vi "CPCI_fifo.vi"(10 "传递队列":refnum<queue>, 11 "notifier":refnum<notifier>) -> ()   [LabVIEW 2012]
uses:
  <vilib>/GPower/VIRegister/Library/Convert/ToBool.vi
  <vilib>/GPower/VIRegister/Library/SubVIs/FindRegisterData.vi
  <vilib>/GPower/VIRegister/Library/SubVIs/ReadSub.vi
  <vilib>/GPower/VIRegister/Library/SubVIs/WriteSub.vi
  <vilib>/GPower/VIRegister/Library/QManager/GetRegisterData.vi
  <vilib>/GPower/Error/Library/SetError.vi
  <vilib>/GPower/Error/Library/FilterCodes.vi
  <vilib>/GPower/Error/Library/Filter/FilterMulti.vi
  <vilib>/GPower/VIRegister/Library/QManager/QManagerAction.vi
  <vilib>/GPower/Error/Library/ErrorType.vi
  <vilib>/GPower/Error/Library/SplitAppended.vi
  <vilib>/GPower/Error/Library/SubVIs/ExplanationToError.vi
  <vilib>/GPower/VIRegister/Library/QManager/GetQName.vi
  <vilib>/GPower/VIRegister/Library/QManager/StartQManager.vi
  <vilib>/Utility/error.llb/Trim Whitespace.vi
  <vilib>/dlg_ctls.llb/Space Constant.vi
  <vilib>/Utility/error.llb/Error Code Database.vi
  <vilib>/GPower/Error/Library/SubVIs/SetStatus.vi
  <vilib>/GPower/Error/Library/AppendErrors.vi
  <vilib>/GPower/Error/Library/Append/AppendSingle.vi
  write32.vi
  write8.vi
  Based_on/BSCT Automation123/BSCT_BasicFunctions/BSCT_BasicFunctions.lvlib
  <vilib>/GPower/VIRegister/VIRegister.lvlib
panel:
  out "x+y 2":u32 format="%.0x"
  out "x+y":u32 format="%.0x"
  in  "8路定时配置 2":T1(array[cluster])=[[{"mode2_set"={"mode2_set01"=0, "mode2_set02"=0, "mode2_set03"=0, "mode2_set04"=0, "mode2_set05"=0, "mode2_set06"=0, "mode2_set07"=0, "mode2_set08"=0, "mode2_set09"=0, "mode2_set10"=0, "mode2_set11"=0, "mode2_set12"=0}, "mode2_t"={"mode2_t01"=0, "mode2_t02"=20, "mode2_t03"=30, "mode2_t04"=0, "mode2_t05"=0, "mode2_t06"=0, "mode2_t07"=0, "mode2_t08"=0, "mode2_t09"=0, "mode2_t10"=0, "mode2_t11"=0, "mode2_t12"=0}, "mode2_cmd_addr"={"mode2_cmd_addr01"=0, "mode2_cmd_addr02"=128, "mode2_cmd_addr03"=256, "mode2_cmd_addr04"=0, "mode2_cmd_addr05"=0, "mode2_cmd_addr06"=0, "mode2_cmd_addr07"=0, "mode2_cmd_addr08"=0, "mode2_cmd_addr09"=0, "mode2_cmd_addr10"=0, "mode2_cmd_addr11"=0, "mode2_cmd_addr12"=0}, "mode2_ cmd_len"={"mode2_ cmd_len01"=20, "mode2_ cmd_len02"=0, "mode2_ cmd_len03"=0, "mode2_ cmd_len04"=0, "mode2_ cmd_len05"=0, "mode2_ cmd_len06"=0, "mode2_ cmd_len07"=0, "mode2_ cmd_len08"=0, "mode2_ cmd_len09"=0, "mode2_ cmd_len10"=0, "mode2_ cmd_len11"=0, "mode2_ cmd_len12"=0}, "mode2_ack_addr"={"mode2_ack_addr01"=0, "mode2_ack_addr02"=128, "mode2_ack_addr03"=256, "mode2_ack_addr04"=0, "mode2_ack_addr05"=0, "mode2_ack_addr06"=0, "mode2_ack_addr07"=0, "mode2_ack_addr08"=0, "mode2_ack_addr09"=0, "mode2_ack_addr10"=0, "mode2_ack_addr11"=0, "mode2_ack_addr12"=0}, "mode2_ack_len"={"mode2_ack_len01"=0, "mode2_ack_len02"=0, "mode2_ack_len03"=0, "mode2_ack_len04"=0, "mode2_ack_len05"=0, "mode2_ack_len06"=0, "mode2_ack_len07"=0, "mode2_ack_len08"=0, "mode2_ack_len09"=0, "mode2_ack_len10"=0, "mode2_ack_len11"=0, "mode2_ack_len12"=0}, "mode2_period"={"mode2_period"=9}}, {"mode2_set"={"mode2_set01"=0, "mode2_set02"=0, "mode2_set03"=0, "mode2_set04"=0, "mode2_set05"=0, "mode2_set06"=0, "mode2_set07"=0, "mode2_set08"=0, "mode2_set09"=0, "mode2_set10"=0, "mode2_set11"=0, "mode2_set12"=0}, "mode2_t"={"mode2_t01"=0, "mode2_t02"=20, "mode2_t03"=30, "mode2_t04"=0, "mode2_t05"=0, "mode2_t06"=0, "mode2_t07"=0, "mode2_t08"=0, "mode2_t09"=0, "mode2_t10"=0, "mode2_t11"=0, "mode2_t12"=0}, "mode2_cmd_addr"={"mode2_cmd_addr01"=0, "mode2_cmd_addr02"=128, "mode2_cmd_addr03"=256, "mode2_cmd_addr04"=0, "mode2_cmd_addr05"=0, "mode2_cmd_addr06"=0, "mode2_cmd_addr07"=0, "mode2_cmd_addr08"=0, "mode2_cmd_addr09"=0, "mode2_cmd_addr10"=0, "mode2_cmd_addr11"=0, "mode2_cmd_addr12"=0}, "mode2_ cmd_len"={"mode2_ cmd_len01"=20, "mode2_ cmd_len02"=0, "mode2_ cmd_len03"=0, "mode2_ cmd_len04"=0, "mode2_ cmd_len05"=0, "mode2_ cmd_len06"=0, "mode2_ cmd_len07"=0, "mode2_ cmd_len08"=0, "mode2_ cmd_len09"=0, "mode2_ cmd_len10"=0, "mode2_ cmd_len11"=0, "mode2_ cmd_len12"=0}, "mode2_ack_addr"={"mode2_ack_addr01"=0, "mode2_ack_addr02"=128, "mode2_ack_addr03"=256, "mode2_ack_addr04"=0, "mode2_ack_addr05"=0, "mode2_ack_addr06"=0, "mode2_ack_addr07"=0, "mode2_ack_addr08"=0, "mode2_ack_addr09"=0, "mode2_ack_addr10"=0, "mode2_ack_addr11"=0, "mode2_ack_addr12"=0}, "mode2_ack_len"={"mode2_ack_len01"=0, "mode2_ack_len02"=0, "mode2_ack_len03"=0, "mode2_ack_len04"=0, "mode2_ack_len05"=0, "mode2_ack_len06"=0, "mode2_ack_len07"=0, "mode2_ack_len08"=0, "mode2_ack_len09"=0, "mode2_ack_len10"=0, "mode2_ack_len11"=0, "mode2_ack_len12"=0}, "mode2_period"={"mode2_period"=9}}, {"mode2_set"={"mode2_set01"=0, "mode2_set02"=0, "mode2_set03"=0, "mode2_set04"=0, "mode2_set05"=0, "mode2_set06"=0, "mode2_set07"=0, "mode2_set08"=0, "mode2_set09"=0, "mode2_set10"=0, "mode2_set11"=0, "mode2_set12"=0}, "mode2_t"={"mode2_t01"=0, "mode2_t02"=10, "mode2_t03"=20, "mode2_t04"=0, "mode2_t05"=0, "mode2_t06"=0, "mode2_t07"=0, "mode2_t08"=0, "mode2_t09"=0, "mode2_t10"=0, "mode2_t11"=0, "mode2_t12"=0}, "mode2_cmd_addr"={"mode2_cmd_addr01"=0, "mode2_cmd_addr02"=128, "mode2_cmd_addr03"=256, "mode2_cmd_addr04"=0, "mode2_cmd_addr05"=0, "mode2_cmd_addr06"=0, "mode2_cmd_addr07"=0, "mode2_cmd_addr08"=0, "mode2_cmd_addr09"=0, "mode2_cmd_addr10"=0, "mode2_cmd_addr11"=0, "mode2_cmd_addr12"=0}, "mode2_ cmd_len"={"mode2_ cmd_len01"=0, "mode2_ cmd_len02"=0, "mode2_ cmd_len03"=0, "mode2_ cmd_len04"=0, "mode2_ cmd_len05"=0, "mode2_ cmd_len06"=0, "mode2_ cmd_len07"=0, "mode2_ cmd_len08"=0, "mode2_ cmd_len09"=0, "mode2_ cmd_len10"=0, "mode2_ cmd_len11"=0, "mode2_ cmd_len12"=0}, "mode2_ack_addr"={"mode2_ack_addr01"=0, "mode2_ack_addr02"=128, "mode2_ack_addr03"=256, "mode2_ack_addr04"=0, "mode2_ack_addr05"=0, "mode2_ack_addr06"=0, "mode2_ack_addr07"=0, "mode2_ack_addr08"=0, "mode2_ack_addr09"=0, "mode2_ack_addr10"=0, "mode2_ack_addr11"=0, "mode2_ack_addr12"=0}, "mode2_ack_len"={"mode2_ack_len01"=0, "mode2_ack_len02"=0, "mode2_ack_len03"=0, "mode2_ack_len04"=0, "mode2_ack_len05"=0, "mode2_ack_len06"=0, "mode2_ack_len07"=0, "mode2_ack_len08"=0, "mode2_ack_len09"=0, "mode2_ack_len10"=0, "mode2_ack_len11"=0, "mode2_ack_len12"=0}, "mode2_period"={"mode2_period"=159}}, {"mode2_set"={"mode2_set01"=0, "mode2_set02"=0, "mode2_set03"=0, "mode2_set04"=0, "mode2_set05"=0, "mode2_set06"=0, "mode2_set07"=0, "mode2_set08"=0, "mode2_set09"=0, "mode2_set10"=0, "mode2_set11"=0, "mode2_set12"=0}, "mode2_t"={"mode2_t01"=0, "mode2_t02"=10, "mode2_t03"=20, "mode2_t04"=0, "mode2_t05"=0, "mode2_t06"=0, "mode2_t07"=0, "mode2_t08"=0, "mode2_t09"=0, "mode2_t10"=0, "mode2_t11"=0, "mode2_t12"=0}, "mode2_cmd_addr"={"mode2_cmd_addr01"=0, "mode2_cmd_addr02"=128, "mode2_cmd_addr03"=256, "mode2_cmd_addr04"=0, "mode2_cmd_addr05"=0, "mode2_cmd_addr06"=0, "mode2_cmd_addr07"=0, "mode2_cmd_addr08"=0, "mode2_cmd_addr09"=0, "mode2_cmd_addr10"=0, "mode2_cmd_addr11"=0, "mode2_cmd_addr12"=0}, "mode2_ cmd_len"={"mode2_ cmd_len01"=0, "mode2_ cmd_len02"=0, "mode2_ cmd_len03"=0, "mode2_ cmd_len04"=0, "mode2_ cmd_len05"=0, "mode2_ cmd_len06"=0, "mode2_ cmd_len07"=0, "mode2_ cmd_len08"=0, "mode2_ cmd_len09"=0, "mode2_ cmd_len10"=0, "mode2_ cmd_len11"=0, "mode2_ cmd_len12"=0}, "mode2_ack_addr"={"mode2_ack_addr01"=0, "mode2_ack_addr02"=128, "mode2_ack_addr03"=256, "mode2_ack_addr04"=0, "mode2_ack_addr05"=0, "mode2_ack_addr06"=0, "mode2_ack_addr07"=0, "mode2_ack_addr08"=0, "mode2_ack_addr09"=0, "mode2_ack_addr10"=0, "mode2_ack_addr11"=0, "mode2_ack_addr12"=0}, "mode2_ack_len"={"mode2_ack_len01"=0, "mode2_ack_len02"=0, "mode2_ack_len03"=0, "mode2_ack_len04"=0, "mode2_ack_len05"=0, "mode2_ack_len06"=0, "mode2_ack_len07"=0, "mode2_ack_len08"=0, "mode2_ack_len09"=0, "mode2_ack_len10"=0, "mode2_ack_len11"=0, "mode2_ack_len12"=0}, "mode2_period"={"mode2_period"=159}}, {"mode2_set"={"mode2_set01"=0, "mode2_set02"=0, "mode2_set03"=0, "mode2_set04"=0, "mode2_set05"=0, "mode2_set06"=0, "mode2_set07"=0, "mode2_set08"=0, "mode2_set09"=0, "mode2_set10"=0, "mode2_set11"=0, "mode2_set12"=0}, "mode2_t"={"mode2_t01"=0, "mode2_t02"=0, "mode2_t03"=0, "mode2_t04"=0, "mode2_t05"=0, "mode2_t06"=0, "mode2_t07"=0, "mode2_t08"=0, "mode2_t09"=0, "mode2_t10"=0, "mode2_t11"=0, "mode2_t12"=0}, "mode2_cmd_addr"={"mode2_cmd_addr01"=0, "mode2_cmd_addr02"=0, "mode2_cmd_addr03"=0, "mode2_cmd_addr04"=0, "mode2_cmd_addr05"=0, "mode2_cmd_addr06"=0, "mode2_cmd_addr07"=0, "mode2_cmd_addr08"=0, "mode2_cmd_addr09"=0, "mode2_cmd_addr10"=0, "mode2_cmd_addr11"=0, "mode2_cmd_addr12"=0}, "mode2_ cmd_len"={"mode2_ cmd_len01"=0, "mode2_ cmd_len02"=0, "mode2_ cmd_len03"=0, "mode2_ cmd_len04"=0, "mode2_ cmd_len05"=0, "mode2_ cmd_len06"=0, "mode2_ cmd_len07"=0, "mode2_ cmd_len08"=0, "mode2_ cmd_len09"=0, "mode2_ cmd_len10"=0, "mode2_ cmd_len11"=0, "mode2_ cmd_len12"=0}, "mode2_ack_addr"={"mode2_ack_addr01"=0, "mode2_ack_addr02"=0, "mode2_ack_addr03"=0, "mode2_ack_addr04"=0, "mode2_ack_addr05"=0, "mode2_ack_addr06"=0, "mode2_ack_addr07"=0, "mode2_ack_addr08"=0, "mode2_ack_addr09"=0, "mode2_ack_addr10"=0, "mode2_ack_addr11"=0, "mode2_ack_addr12"=0}, "mode2_ack_len"={"mode2_ack_len01"=0, "mode2_ack_len02"=0, "mode2_ack_len03"=0, "mode2_ack_len04"=0, "mode2_ack_len05"=0, "mode2_ack_len06"=0, "mode2_ack_len07"=0, "mode2_ack_len08"=0, "mode2_ack_len09"=0, "mode2_ack_len10"=0, "mode2_ack_len11"=0, "mode2_ack_len12"=0}, "mode2_period"={"mode2_period"=0}}, {"mode2_set"={"mode2_set01"=0, "mode2_set02"=0, "mode2_set03"=0, "mode2_set04"=0, "mode2_set05"=0, "mode2_set06"=0, "mode2_set07"=0, "mode2_set08"=0, "mode2_set09"=0, "mode2_set10"=0, "mode2_set11"=0, "mode2_set12"=0}, "mode2_t"={"mode2_t01"=0, "mode2_t02"=0, "mode2_t03"=0, "mode2_t04"=0, "mode2_t05"=0, "mode2_t06"=0, "mode2_t07"=0, "mode2_t08"=0, "mode2_t09"=0, "mode2_t10"=0, "mode2_t11"=0, "mode2_t12"=0}, "mode2_cmd_addr"={"mode2_cmd_addr01"=0, "mode2_cmd_addr02"=0, "mode2_cmd_addr03"=0, "mode2_cmd_addr04"=0, "mode2_cmd_addr05"=0, "mode2_cmd_addr06"=0, "mode2_cmd_addr07"=0, "mode2_cmd_addr08"=0, "mode2_cmd_addr09"=0, "mode2_cmd_addr10"=0, "mode2_cmd_addr11"=0, "mode2_cmd_addr12"=0}, "mode2_ cmd_len"={"mode2_ cmd_len01"=0, "mode2_ cmd_len02"=0, "mode2_ cmd_len03"=0, "mode2_ cmd_len04"=0, "mode2_ cmd_len05"=0, "mode2_ cmd_len06"=0, "mode2_ cmd_len07"=0, "mode2_ cmd_len08"=0, "mode2_ cmd_len09"=0, "mode2_ cmd_len10"=0, "mode2_ cmd_len11"=0, "mode2_ cmd_len12"=0}, "mode2_ack_addr"={"mode2_ack_addr01"=0, "mode2_ack_addr02"=0, "mode2_ack_addr03"=0, "mode2_ack_addr04"=0, "mode2_ack_addr05"=0, "mode2_ack_addr06"=0, "mode2_ack_addr07"=0, "mode2_ack_addr08"=0, "mode2_ack_addr09"=0, "mode2_ack_addr10"=0, "mode2_ack_addr11"=0, "mode2_ack_addr12"=0}, "mode2_ack_len"={"mode2_ack_len01"=0, "mode2_ack_len02"=0, "mode2_ack_len03"=0, "mode2_ack_len04"=0, "mode2_ack_len05"=0, "mode2_ack_len06"=0, "mode2_ack_len07"=0, "mode2_ack_len08"=0, "mode2_ack_len09"=0, "mode2_ack_len10"=0, "mode2_ack_len11"=0, "mode2_ack_len12"=0}, "mode2_period"={"mode2_period"=0}}, {"mode2_set"={"mode2_set01"=0, "mode2_set02"=0, "mode2_set03"=0, "mode2_set04"=0, "mode2_set05"=0, "mode2_set06"=0, "mode2_set07"=0, "mode2_set08"=0, "mode2_set09"=0, "mode2_set10"=0, "mode2_set11"=0, "mode2_set12"=0}, "mode2_t"={"mode2_t01"=0, "mode2_t02"=0, "mode2_t03"=0, "mode2_t04"=0, "mode2_t05"=0, "mode2_t06"=0, "mode2_t07"=0, "mode2_t08"=0, "mode2_t09"=0, "mode2_t10"=0, "mode2_t11"=0, "mode2_t12"=0}, "mode2_cmd_addr"={"mode2_cmd_addr01"=0, "mode2_cmd_addr02"=0, "mode2_cmd_addr03"=0, "mode2_cmd_addr04"=0, "mode2_cmd_addr05"=0, "mode2_cmd_addr06"=0, "mode2_cmd_addr07"=0, "mode2_cmd_addr08"=0, "mode2_cmd_addr09"=0, "mode2_cmd_addr10"=0, "mode2_cmd_addr11"=0, "mode2_cmd_addr12"=0}, "mode2_ cmd_len"={"mode2_ cmd_len01"=0, "mode2_ cmd_len02"=0, "mode2_ cmd_len03"=0, "mode2_ cmd_len04"=0, "mode2_ cmd_len05"=0, "mode2_ cmd_len06"=0, "mode2_ cmd_len07"=0, "mode2_ cmd_len08"=0, "mode2_ cmd_len09"=0, "mode2_ cmd_len10"=0, "mode2_ cmd_len11"=0, "mode2_ cmd_len12"=0}, "mode2_ack_addr"={"mode2_ack_addr01"=0, "mode2_ack_addr02"=0, "mode2_ack_addr03"=0, "mode2_ack_addr04"=0, "mode2_ack_addr05"=0, "mode2_ack_addr06"=0, "mode2_ack_addr07"=0, "mode2_ack_addr08"=0, "mode2_ack_addr09"=0, "mode2_ack_addr10"=0, "mode2_ack_addr11"=0, "mode2_ack_addr12"=0}, "mode2_ack_len"={"mode2_ack_len01"=0, "mode2_ack_len02"=0, "mode2_ack_len03"=0, "mode2_ack_len04"=0, "mode2_ack_len05"=0, "mode2_ack_len06"=0, "mode2_ack_len07"=0, "mode2_ack_len08"=0, "mode2_ack_len09"=0, "mode2_ack_len10"=0, "mode2_ack_len11"=0, "mode2_ack_len12"=0}, "mode2_period"={"mode2_period"=0}}, {"mode2_set"={"mode2_set01"=0, "mode2_set02"=0, "mode2_set03"=0, "mode2_set04"=0, "mode2_set05"=0, "mode2_set06"=0, "mode2_set07"=0, "mode2_set08"=0, "mode2_set09"=0, "mode2_set10"=0, "mode2_set11"=0, "mode2_set12"=0}, "mode2_t"={"mode2_t01"=0, "mode2_t02"=0, "mode2_t03"=0, "mode2_t04"=0, "mode2_t05"=0, "mode2_t06"=0, "mode2_t07"=0, "mode2_t08"=0, "mode2_t09"=0, "mode2_t10"=0, "mode2_t11"=0, "mode2_t12"=0}, "mode2_cmd_addr"={"mode2_cmd_addr01"=0, "mode2_cmd_addr02"=0, "mode2_cmd_addr03"=0, "mode2_cmd_addr04"=0, "mode2_cmd_addr05"=0, "mode2_cmd_addr06"=0, "mode2_cmd_addr07"=0, "mode2_cmd_addr08"=0, "mode2_cmd_addr09"=0, "mode2_cmd_addr10"=0, "mode2_cmd_addr11"=0, "mode2_cmd_addr12"=0}, "mode2_ cmd_len"={"mode2_ cmd_len01"=0, "mode2_ cmd_len02"=0, "mode2_ cmd_len03"=0, "mode2_ cmd_len04"=0, "mode2_ cmd_len05"=0, "mode2_ cmd_len06"=0, "mode2_ cmd_len07"=0, "mode2_ cmd_len08"=0, "mode2_ cmd_len09"=0, "mode2_ cmd_len10"=0, "mode2_ cmd_len11"=0, "mode2_ cmd_len12"=0}, "mode2_ack_addr"={"mode2_ack_addr01"=0, "mode2_ack_addr02"=0, "mode2_ack_addr03"=0, "mode2_ack_addr04"=0, "mode2_ack_addr05"=0, "mode2_ack_addr06"=0, "mode2_ack_addr07"=0, "mode2_ack_addr08"=0, "mode2_ack_addr09"=0, "mode2_ack_addr10"=0, "mode2_ack_addr11"=0, "mode2_ack_addr12"=0}, "mode2_ack_len"={"mode2_ack_len01"=0, "mode2_ack_len02"=0, "mode2_ack_len03"=0, "mode2_ack_len04"=0, "mode2_ack_len05"=0, "mode2_ack_len06"=0, "mode2_ack_len07"=0, "mode2_ack_len08"=0, "mode2_ack_len09"=0, "mode2_ack_len10"=0, "mode2_ack_len11"=0, "mode2_ack_len12"=0}, "mode2_period"={"mode2_period"=0}}], [{"mode2_set"={"mode2_set01"=0, "mode2_set02"=0, "mode2_set03"=0, "mode2_set04"=0, "mode2_set05"=0, "mode2_set06"=0, "mode2_set07"=0, "mode2_set08"=0, "mode2_set09"=0, "mode2_set10"=0, "mode2_set11"=0, "mode2_set12"=0}, "mode2_t"={"mode2_t01"=200, "mode2_t02"=0, "mode2_t03"=0, "mode2_t04"=0, "mode2_t05"=0, "mode2_t06"=0, "mode2_t07"=0, "mode2_t08"=0, "mode2_t09"=0, "mode2_t10"=0, "mode2_t11"=0, "mode2_t12"=0}, "mode2_cmd_addr"={"mode2_cmd_addr01"=0, "mode2_cmd_addr02"=0, "mode2_cmd_addr03"=0, "mode2_cmd_addr04"=0, "mode2_cmd_addr05"=0, "mode2_cmd_addr06"=0, "mode2_cmd_addr07"=0, "mode2_cmd_addr08"=0, "mode2_cmd_addr09"=0, "mode2_cmd_addr10"=0, "mode2_cmd_addr11"=0, "mode2_cmd_addr12"=0}, "mode2_ cmd_len"={"mode2_ cmd_len01"=218, "mode2_ cmd_len02"=0, "mode2_ cmd_len03"=0, "mode2_ cmd_len04"=0, "mode2_ cmd_len05"=0, "mode2_ cmd_len06"=0, "mode2_ cmd_len07"=0, "mode2_ cmd_len08"=0, "mode2_ cmd_len09"=0, "mode2_ cmd_len10"=0, "mode2_ cmd_len11"=0, "mode2_ cmd_len12"=0}, "mode2_ack_addr"={"mode2_ack_addr01"=0, "mode2_ack_addr02"=0, "mode2_ack_addr03"=0, "mode2_ack_addr04"=0, "mode2_ack_addr05"=0, "mode2_ack_addr06"=0, "mode2_ack_addr07"=0, "mode2_ack_addr08"=0, "mode2_ack_addr09"=0, "mode2_ack_addr10"=0, "mode2_ack_addr11"=0, "mode2_ack_addr12"=0}, "mode2_ack_len"={"mode2_ack_len01"=0, "mode2_ack_len02"=0, "mode2_ack_len03"=0, "mode2_ack_len04"=0, "mode2_ack_len05"=0, "mode2_ack_len06"=0, "mode2_ack_len07"=0, "mode2_ack_len08"=0, "mode2_ack_len09"=0, "mode2_ack_len10"=0, "mode2_ack_len11"=0, "mode2_ack_len12"=0}, "mode2_period"={"mode2_period"=1000}}, {"mode2_set"={"mode2_set01"=0, "mode2_set02"=0, "mode2_set03"=0, "mode2_set04"=0, "mode2_set05"=0, "mode2_set06"=0, "mode2_set07"=0, "mode2_set08"=0, "mode2_set09"=0, "mode2_set10"=0, "mode2_set11"=0, "mode2_set12"=0}, "mode2_t"={"mode2_t01"=0, "mode2_t02"=0, "mode2_t03"=0, "mode2_t04"=0, "mode2_t05"=0, "mode2_t06"=0, "mode2_t07"=0, "mode2_t08"=0, "mode2_t09"=0, "mode2_t10"=0, "mode2_t11"=0, "mode2_t12"=0}, "mode2_cmd_addr"={"mode2_cmd_addr01"=0, "mode2_cmd_addr02"=0, "mode2_cmd_addr03"=0, "mode2_cmd_addr04"=0, "mode2_cmd_addr05"=0, "mode2_cmd_addr06"=0, "mode2_cmd_addr07"=0, "mode2_cmd_addr08"=0, "mode2_cmd_addr09"=0, "mode2_cmd_addr10"=0, "mode2_cmd_addr11"=0, "mode2_cmd_addr12"=0}, "mode2_ cmd_len"={"mode2_ cmd_len01"=0, "mode2_ cmd_len02"=0, "mode2_ cmd_len03"=0, "mode2_ cmd_len04"=0, "mode2_ cmd_len05"=0, "mode2_ cmd_len06"=0, "mode2_ cmd_len07"=0, "mode2_ cmd_len08"=0, "mode2_ cmd_len09"=0, "mode2_ cmd_len10"=0, "mode2_ cmd_len11"=0, "mode2_ cmd_len12"=0}, "mode2_ack_addr"={"mode2_ack_addr01"=0, "mode2_ack_addr02"=0, "mode2_ack_addr03"=0, "mode2_ack_addr04"=0, "mode2_ack_addr05"=0, "mode2_ack_addr06"=0, "mode2_ack_addr07"=0, "mode2_ack_addr08"=0, "mode2_ack_addr09"=0, "mode2_ack_addr10"=0, "mode2_ack_addr11"=0, "mode2_ack_addr12"=0}, "mode2_ack_len"={"mode2_ack_len01"=0, "mode2_ack_len02"=0, "mode2_ack_len03"=0, "mode2_ack_len04"=0, "mode2_ack_len05"=0, "mode2_ack_len06"=0, "mode2_ack_len07"=0, "mode2_ack_len08"=0, "mode2_ack_len09"=0, "mode2_ack_len10"=0, "mode2_ack_len11"=0, "mode2_ack_len12"=0}, "mode2_period"={"mode2_period"=1000}}, {"mode2_set"={"mode2_set01"=0, "mode2_set02"=0, "mode2_set03"=0, "mode2_set04"=0, "mode2_set05"=0, "mode2_set06"=0, "mode2_set07"=0, "mode2_set08"=0, "mode2_set09"=0, "mode2_set10"=0, "mode2_set11"=0, "mode2_set12"=0}, "mode2_t"={"mode2_t01"=200, "mode2_t02"=0, "mode2_t03"=0, "mode2_t04"=0, "mode2_t05"=0, "mode2_t06"=0, "mode2_t07"=0, "mode2_t08"=0, "mode2_t09"=0, "mode2_t10"=0, "mode2_t11"=0, "mode2_t12"=0}, "mode2_cmd_addr"={"mode2_cmd_addr01"=0, "mode2_cmd_addr02"=0, "mode2_cmd_addr03"=0, "mode2_cmd_addr04"=0, "mode2_cmd_addr05"=0, "mode2_cmd_addr06"=0, "mode2_cmd_addr07"=0, "mode2_cmd_addr08"=0, "mode2_cmd_addr09"=0, "mode2_cmd_addr10"=0, "mode2_cmd_addr11"=0, "mode2_cmd_addr12"=0}, "mode2_ cmd_len"={"mode2_ cmd_len01"=218, "mode2_ cmd_len02"=0, "mode2_ cmd_len03"=0, "mode2_ cmd_len04"=0, "mode2_ cmd_len05"=0, "mode2_ cmd_len06"=0, "mode2_ cmd_len07"=0, "mode2_ cmd_len08"=0, "mode2_ cmd_len09"=0, "mode2_ cmd_len10"=0, "mode2_ cmd_len11"=0, "mode2_ cmd_len12"=0}, "mode2_ack_addr"={"mode2_ack_addr01"=0, "mode2_ack_addr02"=0, "mode2_ack_addr03"=0, "mode2_ack_addr04"=0, "mode2_ack_addr05"=0, "mode2_ack_addr06"=0, "mode2_ack_addr07"=0, "mode2_ack_addr08"=0, "mode2_ack_addr09"=0, "mode2_ack_addr10"=0, "mode2_ack_addr11"=0, "mode2_ack_addr12"=0}, "mode2_ack_len"={"mode2_ack_len01"=0, "mode2_ack_len02"=0, "mode2_ack_len03"=0, "mode2_ack_len04"=0, "mode2_ack_len05"=0, "mode2_ack_len06"=0, "mode2_ack_len07"=0, "mode2_ack_len08"=0, "mode2_ack_len09"=0, "mode2_ack_len10"=0, "mode2_ack_len11"=0, "mode2_ack_len12"=0}, "mode2_period"={"mode2_period"=1000}}, {"mode2_set"={"mode2_set01"=0, "mode2_set02"=0, "mode2_set03"=0, "mode2_set04"=0, "mode2_set05"=0, "mode2_set06"=0, "mode2_set07"=0, "mode2_set08"=0, "mode2_set09"=0, "mode2_set10"=0, "mode2_set11"=0, "mode2_set12"=0}, "mode2_t"={"mode2_t01"=0, "mode2_t02"=0, "mode2_t03"=0, "mode2_t04"=0, "mode2_t05"=0, "mode2_t06"=0, "mode2_t07"=0, "mode2_t08"=0, "mode2_t09"=0, "mode2_t10"=0, "mode2_t11"=0, "mode2_t12"=0}, "mode2_cmd_addr"={"mode2_cmd_addr01"=0, "mode2_cmd_addr02"=0, "mode2_cmd_addr03"=0, "mode2_cmd_addr04"=0, "mode2_cmd_addr05"=0, "mode2_cmd_addr06"=0, "mode2_cmd_addr07"=0, "mode2_cmd_addr08"=0, "mode2_cmd_addr09"=0, "mode2_cmd_addr10"=0, "mode2_cmd_addr11"=0, "mode2_cmd_addr12"=0}, "mode2_ cmd_len"={"mode2_ cmd_len01"=0, "mode2_ cmd_len02"=0, "mode2_ cmd_len03"=0, "mode2_ cmd_len04"=0, "mode2_ cmd_len05"=0, "mode2_ cmd_len06"=0, "mode2_ cmd_len07"=0, "mode2_ cmd_len08"=0, "mode2_ cmd_len09"=0, "mode2_ cmd_len10"=0, "mode2_ cmd_len11"=0, "mode2_ cmd_len12"=0}, "mode2_ack_addr"={"mode2_ack_addr01"=0, "mode2_ack_addr02"=0, "mode2_ack_addr03"=0, "mode2_ack_addr04"=0, "mode2_ack_addr05"=0, "mode2_ack_addr06"=0, "mode2_ack_addr07"=0, "mode2_ack_addr08"=0, "mode2_ack_addr09"=0, "mode2_ack_addr10"=0, "mode2_ack_addr11"=0, "mode2_ack_addr12"=0}, "mode2_ack_len"={"mode2_ack_len01"=0, "mode2_ack_len02"=0, "mode2_ack_len03"=0, "mode2_ack_len04"=0, "mode2_ack_len05"=0, "mode2_ack_len06"=0, "mode2_ack_len07"=0, "mode2_ack_len08"=0, "mode2_ack_len09"=0, "mode2_ack_len10"=0, "mode2_ack_len11"=0, "mode2_ack_len12"=0}, "mode2_period"={"mode2_period"=1000}}, {"mode2_set"={"mode2_set01"=2, "mode2_set02"=0, "mode2_set03"=0, "mode2_set04"=0, "mode2_set05"=0, "mode2_set06"=0, "mode2_set07"=0, "mode2_set08"=0, "mode2_set09"=0, "mode2_set10"=0, "mode2_set11"=0, "mode2_set12"=0}, "mode2_t"={"mode2_t01"=200, "mode2_t02"=0, "mode2_t03"=0, "mode2_t04"=0, "mode2_t05"=0, "mode2_t06"=0, "mode2_t07"=0, "mode2_t08"=0, "mode2_t09"=0, "mode2_t10"=0, "mode2_t11"=0, "mode2_t12"=0}, "mode2_cmd_addr"={"mode2_cmd_addr01"=0, "mode2_cmd_addr02"=0, "mode2_cmd_addr03"=0, "mode2_cmd_addr04"=0, "mode2_cmd_addr05"=0, "mode2_cmd_addr06"=0, "mode2_cmd_addr07"=0, "mode2_cmd_addr08"=0, "mode2_cmd_addr09"=0, "mode2_cmd_addr10"=0, "mode2_cmd_addr11"=0, "mode2_cmd_addr12"=0}, "mode2_ cmd_len"={"mode2_ cmd_len01"=218, "mode2_ cmd_len02"=0, "mode2_ cmd_len03"=0, "mode2_ cmd_len04"=0, "mode2_ cmd_len05"=0, "mode2_ cmd_len06"=0, "mode2_ cmd_len07"=0, "mode2_ cmd_len08"=0, "mode2_ cmd_len09"=0, "mode2_ cmd_len10"=0, "mode2_ cmd_len11"=0, "mode2_ cmd_len12"=0}, "mode2_ack_addr"={"mode2_ack_addr01"=0, "mode2_ack_addr02"=0, "mode2_ack_addr03"=0, "mode2_ack_addr04"=0, "mode2_ack_addr05"=0, "mode2_ack_addr06"=0, "mode2_ack_addr07"=0, "mode2_ack_addr08"=0, "mode2_ack_addr09"=0, "mode2_ack_addr10"=0, "mode2_ack_addr11"=0, "mode2_ack_addr12"=0}, "mode2_ack_len"={"mode2_ack_len01"=0, "mode2_ack_len02"=0, "mode2_ack_len03"=0, "mode2_ack_len04"=0, "mode2_ack_len05"=0, "mode2_ack_len06"=0, "mode2_ack_len07"=0, "mode2_ack_len08"=0, "mode2_ack_len09"=0, "mode2_ack_len10"=0, "mode2_ack_len11"=0, "mode2_ack_len12"=0}, "mode2_period"={"mode2_period"=1000}}, {"mode2_set"={"mode2_set01"=0, "mode2_set02"=0, "mode2_set03"=0, "mode2_set04"=0, "mode2_set05"=0, "mode2_set06"=0, "mode2_set07"=0, "mode2_set08"=0, "mode2_set09"=0, "mode2_set10"=0, "mode2_set11"=0, "mode2_set12"=0}, "mode2_t"={"mode2_t01"=0, "mode2_t02"=0, "mode2_t03"=0, "mode2_t04"=0, "mode2_t05"=0, "mode2_t06"=0, "mode2_t07"=0, "mode2_t08"=0, "mode2_t09"=0, "mode2_t10"=0, "mode2_t11"=0, "mode2_t12"=0}, "mode2_cmd_addr"={"mode2_cmd_addr01"=0, "mode2_cmd_addr02"=0, "mode2_cmd_addr03"=0, "mode2_cmd_addr04"=0, "mode2_cmd_addr05"=0, "mode2_cmd_addr06"=0, "mode2_cmd_addr07"=0, "mode2_cmd_addr08"=0, "mode2_cmd_addr09"=0, "mode2_cmd_addr10"=0, "mode2_cmd_addr11"=0, "mode2_cmd_addr12"=0}, "mode2_ cmd_len"={"mode2_ cmd_len01"=0, "mode2_ cmd_len02"=0, "mode2_ cmd_len03"=0, "mode2_ cmd_len04"=0, "mode2_ cmd_len05"=0, "mode2_ cmd_len06"=0, "mode2_ cmd_len07"=0, "mode2_ cmd_len08"=0, "mode2_ cmd_len09"=0, "mode2_ cmd_len10"=0, "mode2_ cmd_len11"=0, "mode2_ cmd_len12"=0}, "mode2_ack_addr"={"mode2_ack_addr01"=0, "mode2_ack_addr02"=0, "mode2_ack_addr03"=0, "mode2_ack_addr04"=0, "mode2_ack_addr05"=0, "mode2_ack_addr06"=0, "mode2_ack_addr07"=0, "mode2_ack_addr08"=0, "mode2_ack_addr09"=0, "mode2_ack_addr10"=0, "mode2_ack_addr11"=0, "mode2_ack_addr12"=0}, "mode2_ack_len"={"mode2_ack_len01"=0, "mode2_ack_len02"=0, "mode2_ack_len03"=0, "mode2_ack_len04"=0, "mode2_ack_len05"=0, "mode2_ack_len06"=0, "mode2_ack_len07"=0, "mode2_ack_len08"=0, "mode2_ack_len09"=0, "mode2_ack_len10"=0, "mode2_ack_len11"=0, "mode2_ack_len12"=0}, "mode2_period"={"mode2_period"=1000}}, {"mode2_set"={"mode2_set01"=0, "mode2_set02"=0, "mode2_set03"=0, "mode2_set04"=0, "mode2_set05"=0, "mode2_set06"=0, "mode2_set07"=0, "mode2_set08"=0, "mode2_set09"=0, "mode2_set10"=0, "mode2_set11"=0, "mode2_set12"=0}, "mode2_t"={"mode2_t01"=0, "mode2_t02"=0, "mode2_t03"=0, "mode2_t04"=0, "mode2_t05"=0, "mode2_t06"=0, "mode2_t07"=0, "mode2_t08"=0, "mode2_t09"=0, "mode2_t10"=0, "mode2_t11"=0, "mode2_t12"=0}, "mode2_cmd_addr"={"mode2_cmd_addr01"=0, "mode2_cmd_addr02"=0, "mode2_cmd_addr03"=0, "mode2_cmd_addr04"=0, "mode2_cmd_addr05"=0, "mode2_cmd_addr06"=0, "mode2_cmd_addr07"=0, "mode2_cmd_addr08"=0, "mode2_cmd_addr09"=0, "mode2_cmd_addr10"=0, "mode2_cmd_addr11"=0, "mode2_cmd_addr12"=0}, "mode2_ cmd_len"={"mode2_ cmd_len01"=0, "mode2_ cmd_len02"=0, "mode2_ cmd_len03"=0, "mode2_ cmd_len04"=0, "mode2_ cmd_len05"=0, "mode2_ cmd_len06"=0, "mode2_ cmd_len07"=0, "mode2_ cmd_len08"=0, "mode2_ cmd_len09"=0, "mode2_ cmd_len10"=0, "mode2_ cmd_len11"=0, "mode2_ cmd_len12"=0}, "mode2_ack_addr"={"mode2_ack_addr01"=0, "mode2_ack_addr02"=0, "mode2_ack_addr03"=0, "mode2_ack_addr04"=0, "mode2_ack_addr05"=0, "mode2_ack_addr06"=0, "mode2_ack_addr07"=0, "mode2_ack_addr08"=0, "mode2_ack_addr09"=0, "mode2_ack_addr10"=0, "mode2_ack_addr11"=0, "mode2_ack_addr12"=0}, "mode2_ack_len"={"mode2_ack_len01"=0, "mode2_ack_len02"=0, "mode2_ack_len03"=0, "mode2_ack_len04"=0, "mode2_ack_len05"=0, "mode2_ack_len06"=0, "mode2_ack_len07"=0, "mode2_ack_len08"=0, "mode2_ack_len09"=0, "mode2_ack_len10"=0, "mode2_ack_len11"=0, "mode2_ack_len12"=0}, "mode2_period"={"mode2_period"=0}}, {"mode2_set"={"mode2_set01"=0, "mode2_set02"=0, "mode2_set03"=0, "mode2_set04"=0, "mode2_set05"=0, "mode2_set06"=0, "mode2_set07"=0, "mode2_set08"=0, "mode2_set09"=0, "mode2_set10"=0, "mode2_set11"=0, "mode2_set12"=0}, "mode2_t"={"mode2_t01"=0, "mode2_t02"=0, "mode2_t03"=0, "mode2_t04"=0, "mode2_t05"=0, "mode2_t06"=0, "mode2_t07"=0, "mode2_t08"=0, "mode2_t09"=0, "mode2_t10"=0, "mode2_t11"=0, "mode2_t12"=0}, "mode2_cmd_addr"={"mode2_cmd_addr01"=0, "mode2_cmd_addr02"=0, "mode2_cmd_addr03"=0, "mode2_cmd_addr04"=0, "mode2_cmd_addr05"=0, "mode2_cmd_addr06"=0, "mode2_cmd_addr07"=0, "mode2_cmd_addr08"=0, "mode2_cmd_addr09"=0, "mode2_cmd_addr10"=0, "mode2_cmd_addr11"=0, "mode2_cmd_addr12"=0}, "mode2_ cmd_len"={"mode2_ cmd_len01"=0, "mode2_ cmd_len02"=0, "mode2_ cmd_len03"=0, "mode2_ cmd_len04"=0, "mode2_ cmd_len05"=0, "mode2_ cmd_len06"=0, "mode2_ cmd_len07"=0, "mode2_ cmd_len08"=0, "mode2_ cmd_len09"=0, "mode2_ cmd_len10"=0, "mode2_ cmd_len11"=0, "mode2_ cmd_len12"=0}, "mode2_ack_addr"={"mode2_ack_addr01"=0, "mode2_ack_addr02"=0, "mode2_ack_addr03"=0, "mode2_ack_addr04"=0, "mode2_ack_addr05"=0, "mode2_ack_addr06"=0, "mode2_ack_addr07"=0, "mode2_ack_addr08"=0, "mode2_ack_addr09"=0, "mode2_ack_addr10"=0, "mode2_ack_addr11"=0, "mode2_ack_addr12"=0}, "mode2_ack_len"={"mode2_ack_len01"=0, "mode2_ack_len02"=0, "mode2_ack_len03"=0, "mode2_ack_len04"=0, "mode2_ack_len05"=0, "mode2_ack_len06"=0, "mode2_ack_len07"=0, "mode2_ack_len08"=0, "mode2_ack_len09"=0, "mode2_ack_len10"=0, "mode2_ack_len11"=0, "mode2_ack_len12"=0}, "mode2_period"={"mode2_period"=0}}]] {"mode2_cmd_addr"."mode2_cmd_addr01" format="%.0x"; "mode2_cmd_addr"."mode2_cmd_addr02" format="%.0x"; "mode2_cmd_addr"."mode2_cmd_addr03" format="%.0x"; "mode2_ack_addr"."mode2_ack_addr02" format="%.0x"; "mode2_ack_addr"."mode2_ack_addr03" format="%.0x"; "mode2_ack_len"."mode2_ack_len01" format="%.0x"; "mode2_ack_len"."mode2_ack_len02" format="%.0x"; "mode2_ack_len"."mode2_ack_len03" format="%.0x"}
  in  "8路通用配置":T2(array[cluster])=[[{"rx_on"=1, " tx_on"=1, "parity"=3, "stop_bit"=1, "baudrate"=434, "sample_ph"=4, "clk_freq"=50000, "rx_ interval"=50, "tx_ interval"=0, "force_tx_low"=0, "rx_ptr_rst"=0, "rx_debug_cnt_clr"=0, "rx_wrong_data_clr"=0}, {"rx_on"=1, " tx_on"=1, "parity"=3, "stop_bit"=1, "baudrate"=434, "sample_ph"=4, "clk_freq"=50000, "rx_ interval"=50, "tx_ interval"=0, "force_tx_low"=0, "rx_ptr_rst"=0, "rx_debug_cnt_clr"=0, "rx_wrong_data_clr"=0}, {"rx_on"=1, " tx_on"=1, "parity"=0, "stop_bit"=0, "baudrate"=108, "sample_ph"=4, "clk_freq"=50000, "rx_ interval"=50, "tx_ interval"=0, "force_tx_low"=0, "rx_ptr_rst"=0, "rx_debug_cnt_clr"=0, "rx_wrong_data_clr"=0}, {"rx_on"=1, " tx_on"=1, "parity"=0, "stop_bit"=0, "baudrate"=108, "sample_ph"=4, "clk_freq"=50000, "rx_ interval"=50, "tx_ interval"=0, "force_tx_low"=0, "rx_ptr_rst"=0, "rx_debug_cnt_clr"=0, "rx_wrong_data_clr"=0}, {"rx_on"=1, " tx_on"=1, "parity"=3, "stop_bit"=0, "baudrate"=434, "sample_ph"=4, "clk_freq"=50000, "rx_ interval"=50, "tx_ interval"=0, "force_tx_low"=0, "rx_ptr_rst"=0, "rx_debug_cnt_clr"=0, "rx_wrong_data_clr"=0}, {"rx_on"=1, " tx_on"=1, "parity"=3, "stop_bit"=0, "baudrate"=434, "sample_ph"=4, "clk_freq"=50000, "rx_ interval"=50, "tx_ interval"=0, "force_tx_low"=0, "rx_ptr_rst"=0, "rx_debug_cnt_clr"=0, "rx_wrong_data_clr"=0}, {"rx_on"=1, " tx_on"=1, "parity"=3, "stop_bit"=0, "baudrate"=434, "sample_ph"=4, "clk_freq"=50000, "rx_ interval"=50, "tx_ interval"=0, "force_tx_low"=0, "rx_ptr_rst"=0, "rx_debug_cnt_clr"=0, "rx_wrong_data_clr"=0}, {"rx_on"=1, " tx_on"=1, "parity"=3, "stop_bit"=0, "baudrate"=434, "sample_ph"=4, "clk_freq"=50000, "rx_ interval"=50, "tx_ interval"=0, "force_tx_low"=0, "rx_ptr_rst"=0, "rx_debug_cnt_clr"=0, "rx_wrong_data_clr"=0}], [{"rx_on"=1, " tx_on"=1, "parity"=3, "stop_bit"=1, "baudrate"=434, "sample_ph"=4, "clk_freq"=50000, "rx_ interval"=50, "tx_ interval"=0, "force_tx_low"=0, "rx_ptr_rst"=0, "rx_debug_cnt_clr"=0, "rx_wrong_data_clr"=0}, {"rx_on"=1, " tx_on"=1, "parity"=3, "stop_bit"=1, "baudrate"=434, "sample_ph"=4, "clk_freq"=50000, "rx_ interval"=50, "tx_ interval"=0, "force_tx_low"=0, "rx_ptr_rst"=0, "rx_debug_cnt_clr"=0, "rx_wrong_data_clr"=0}, {"rx_on"=1, " tx_on"=1, "parity"=3, "stop_bit"=1, "baudrate"=434, "sample_ph"=4, "clk_freq"=50000, "rx_ interval"=50, "tx_ interval"=0, "force_tx_low"=0, "rx_ptr_rst"=0, "rx_debug_cnt_clr"=0, "rx_wrong_data_clr"=0}, {"rx_on"=1, " tx_on"=1, "parity"=3, "stop_bit"=1, "baudrate"=434, "sample_ph"=4, "clk_freq"=50000, "rx_ interval"=50, "tx_ interval"=0, "force_tx_low"=0, "rx_ptr_rst"=0, "rx_debug_cnt_clr"=0, "rx_wrong_data_clr"=0}, {"rx_on"=1, " tx_on"=1, "parity"=3, "stop_bit"=1, "baudrate"=434, "sample_ph"=4, "clk_freq"=50000, "rx_ interval"=50, "tx_ interval"=0, "force_tx_low"=0, "rx_ptr_rst"=0, "rx_debug_cnt_clr"=0, "rx_wrong_data_clr"=0}, {"rx_on"=1, " tx_on"=1, "parity"=3, "stop_bit"=1, "baudrate"=434, "sample_ph"=4, "clk_freq"=50000, "rx_ interval"=50, "tx_ interval"=0, "force_tx_low"=0, "rx_ptr_rst"=0, "rx_debug_cnt_clr"=0, "rx_wrong_data_clr"=0}, {"rx_on"=1, " tx_on"=1, "parity"=3, "stop_bit"=1, "baudrate"=434, "sample_ph"=4, "clk_freq"=50000, "rx_ interval"=50, "tx_ interval"=0, "force_tx_low"=0, "rx_ptr_rst"=0, "rx_debug_cnt_clr"=0, "rx_wrong_data_clr"=0}, {"rx_on"=1, " tx_on"=1, "parity"=3, "stop_bit"=1, "baudrate"=434, "sample_ph"=4, "clk_freq"=50000, "rx_ interval"=50, "tx_ interval"=0, "force_tx_low"=0, "rx_ptr_rst"=0, "rx_debug_cnt_clr"=0, "rx_wrong_data_clr"=0}]]
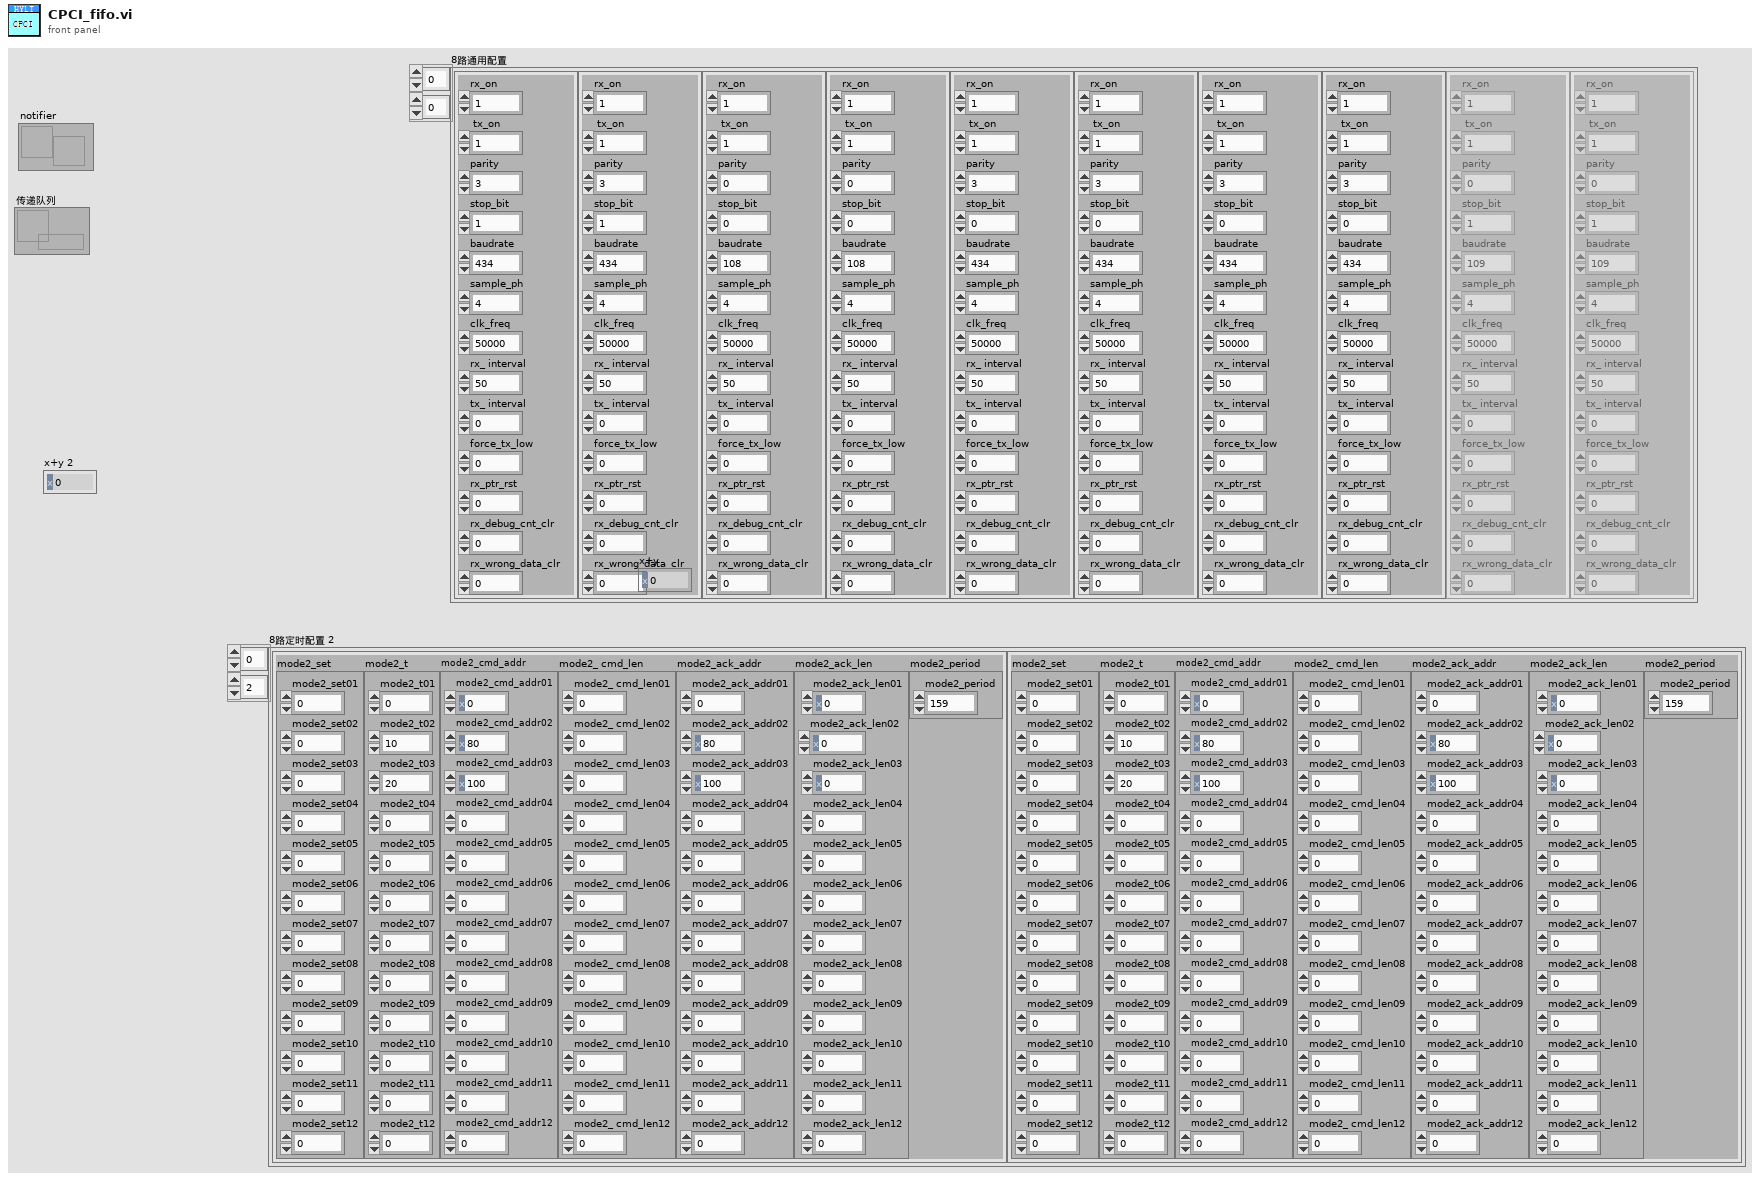
[diagram p1: front panel]
types:
  T1 = cluster{"mode2_set":cluster{"mode2_set01":u8, "mode2_set02":u8, "mode2_set03":u8, "mode2_set04":u8, "mode2_set05":u8, "mode2_set06":u8, "mode2_set07":u8, "mode2_set08":u8, "mode2_set09":u8, "mode2_set10":u8, "mode2_set11":u8, "mode2_set12":u8}, "mode2_t":cluster{"mode2_t01":u16, "mode2_t02":u16, "mode2_t03":u16, "mode2_t04":u16, "mode2_t05":u16, "mode2_t06":u16, "mode2_t07":u16, "mode2_t08":u16, "mode2_t09":u16, "mode2_t10":u16, "mode2_t11":u16, "mode2_t12":u16}, "mode2_cmd_addr":cluster{"mode2_cmd_addr01":u16, "mode2_cmd_addr02":u16, "mode2_cmd_addr03":u16, "mode2_cmd_addr04":u16, "mode2_cmd_addr05":u16, "mode2_cmd_addr06":u16, "mode2_cmd_addr07":u16, "mode2_cmd_addr08":u16, "mode2_cmd_addr09":u16, "mode2_cmd_addr10":u16, "mode2_cmd_addr11":u16, "mode2_cmd_addr12":u16}, "mode2_ cmd_len":cluster{"mode2_ cmd_len01":u16, "mode2_ cmd_len02":u16, "mode2_ cmd_len03":u16, "mode2_ cmd_len04":u16, "mode2_ cmd_len05":u16, "mode2_ cmd_len06":u16, "mode2_ cmd_len07":u16, "mode2_ cmd_len08":u16, "mode2_ cmd_len09":u16, "mode2_ cmd_len10":u16, "mode2_ cmd_len11":u16, "mode2_ cmd_len12":u16}, "mode2_ack_addr":cluster{"mode2_ack_addr01":u16, "mode2_ack_addr02":u16, "mode2_ack_addr03":u16, "mode2_ack_addr04":u16, "mode2_ack_addr05":u16, "mode2_ack_addr06":u16, "mode2_ack_addr07":u16, "mode2_ack_addr08":u16, "mode2_ack_addr09":u16, "mode2_ack_addr10":u16, "mode2_ack_addr11":u16, "mode2_ack_addr12":u16}, "mode2_ack_len":cluster{"mode2_ack_len01":u16, "mode2_ack_len02":u16, "mode2_ack_len03":u16, "mode2_ack_len04":u16, "mode2_ack_len05":u16, "mode2_ack_len06":u16, "mode2_ack_len07":u16, "mode2_ack_len08":u16, "mode2_ack_len09":u16, "mode2_ack_len10":u16, "mode2_ack_len11":u16, "mode2_ack_len12":u16}, "mode2_period":cluster{"mode2_period":u32}}[][]
  T2 = cluster{"rx_on":u8, " tx_on":u8, "parity":u8, "stop_bit":u8, "baudrate":u16, "sample_ph":u16, "clk_freq":u32, "rx_ interval":u16, "tx_ interval":u16, "force_tx_low":u32, "rx_ptr_rst":u8, "rx_debug_cnt_clr":u8, "rx_wrong_data_clr":u16}[][]
  T3 = enum32{"invalid app kind", "Development System", "Run Time System", "Student Edition", "Embedded LabVIEW", "Evaluation", "Custom"}
  T4 = enum32{"Invalid", "Standard", "Closed", "Hidden", "Minimized", "Maximized"}
  T5 = cluster{"Core":cluster{"Current VI Reference":refnum<vi>, "Close Panel on Exit?":bool}, "Your Boolean data":bool, "Your string data":string, "地检1相位":i32, "地检2相位":i32, "millisecond timer value":u32, "VISA资源名称":refnum<visa-resource-name>}
  T6 = cluster{"Current VI Reference":refnum<vi>, "Close Panel on Exit?":bool}
  T7 = cluster{"主份通道选择":enum32{"通道A", "通道B"}, "备份通道选择":enum32{"通道A", "通道B"}}
  T8 = cluster{"Core":cluster{"Current VI Reference":refnum<vi>, "Close Panel on Exit?":bool}, "visa":refnum<visa-resource-name>[], "主份通道选择":enum8{"ChanleA", "ChanelB"}, "备份通道选择":enum8{"ChanleA", "ChanelB"}, "毫秒计时值":u32, "notifier ":refnum<notifier>}
  T9 = cluster{" 数据帧名称":string, " 数据":string, "备用操作符":bool, "起始地址":i32, "读写标志":i32, "长度":i32}
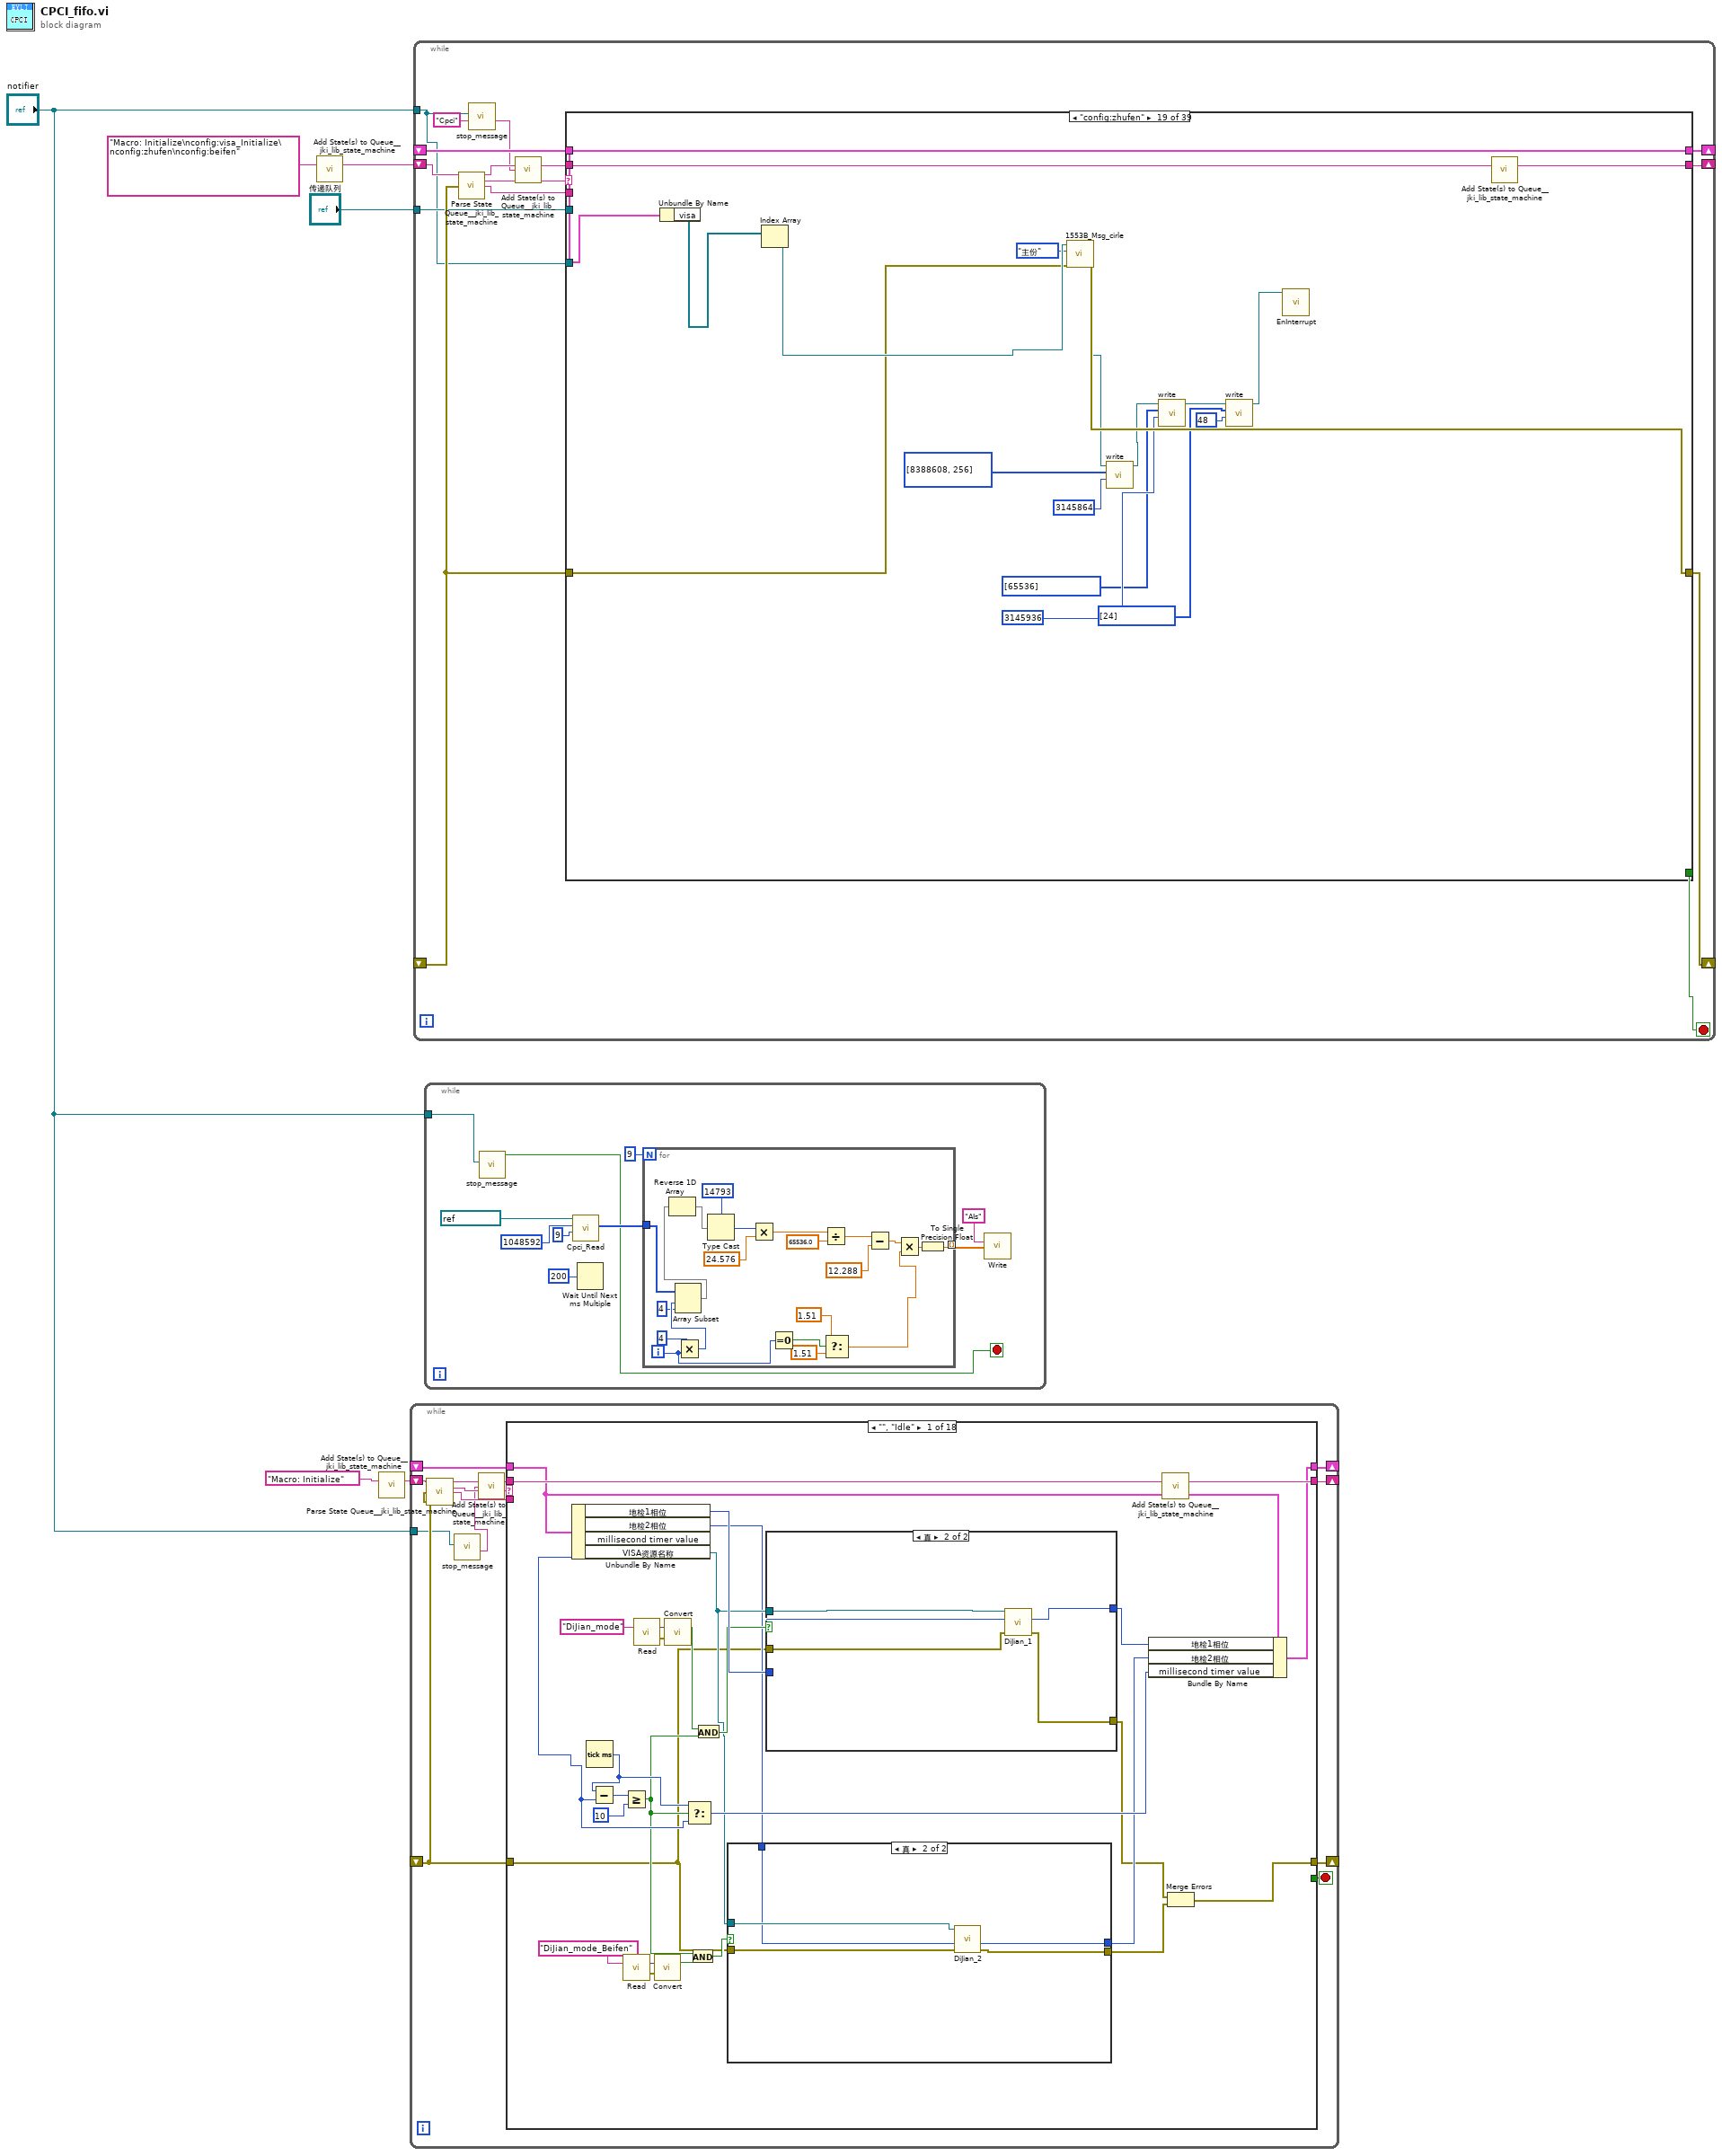
[diagram p0: block diagram]
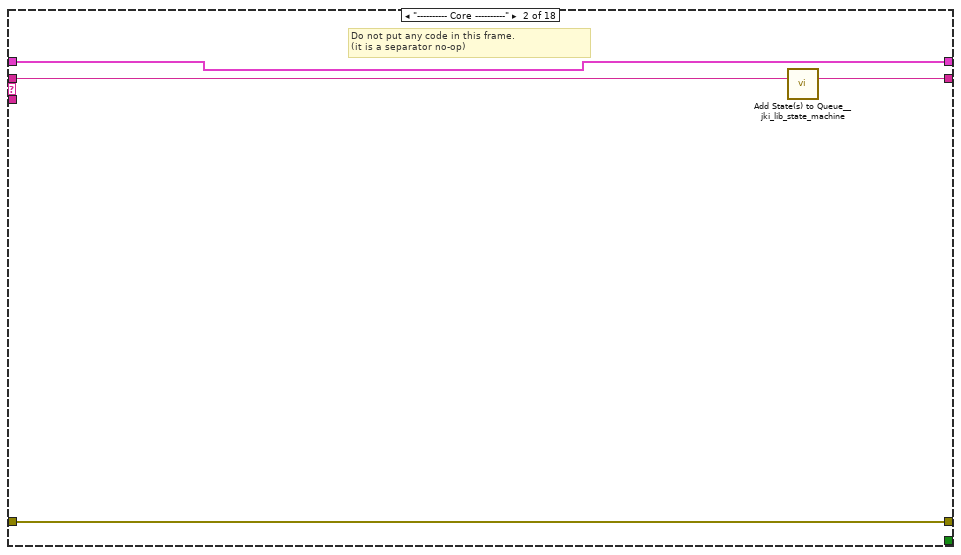
[diagram p4: hidden frame]
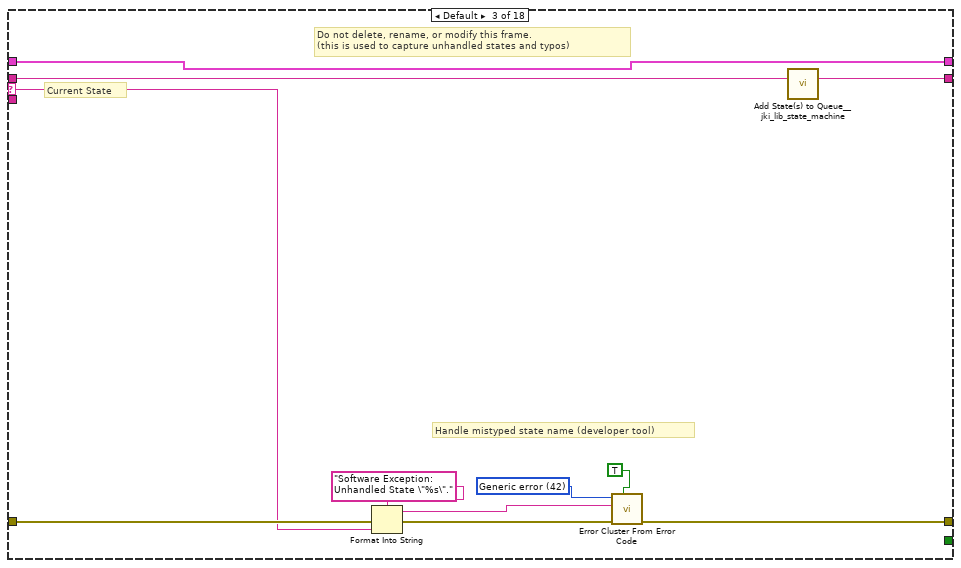
[diagram p5: hidden frame]
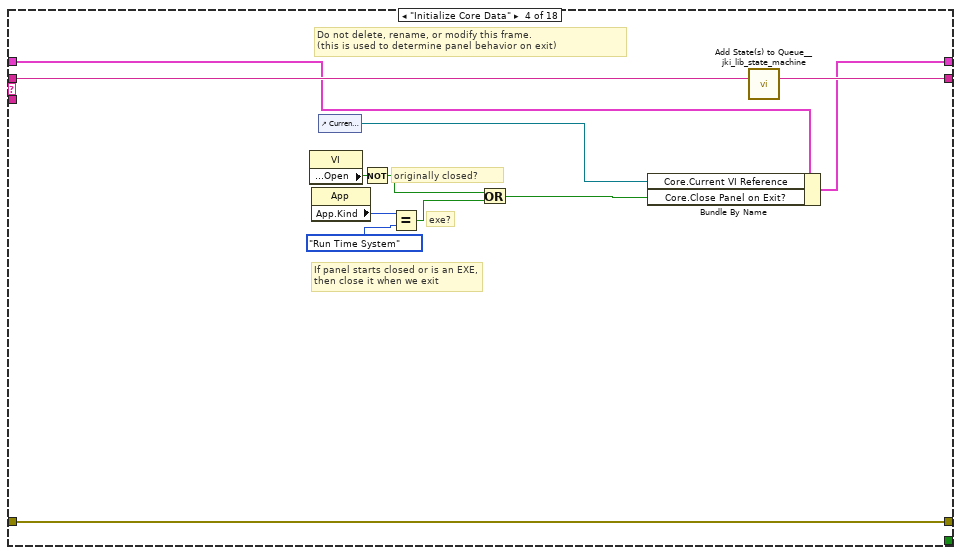
[diagram p6: hidden frame]
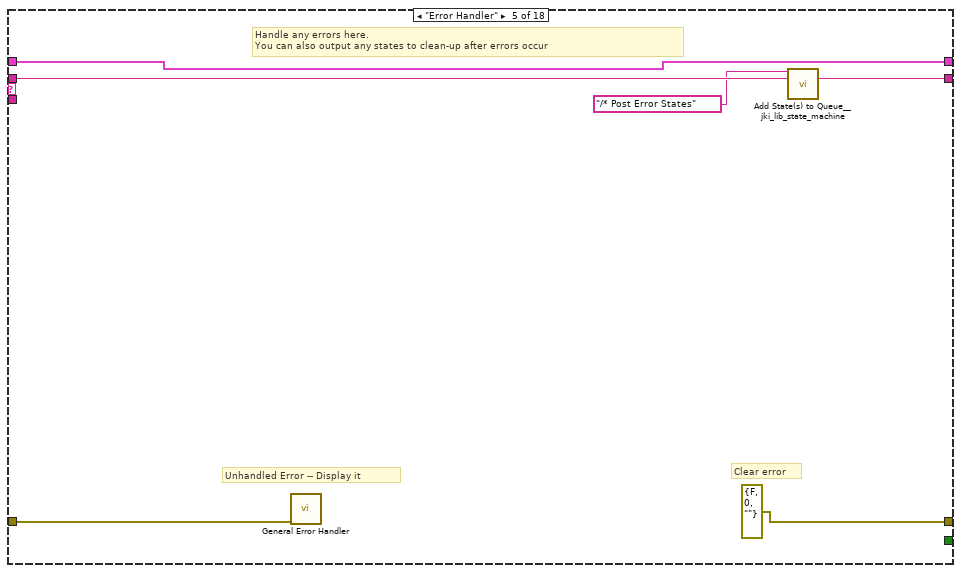
[diagram p7: hidden frame]
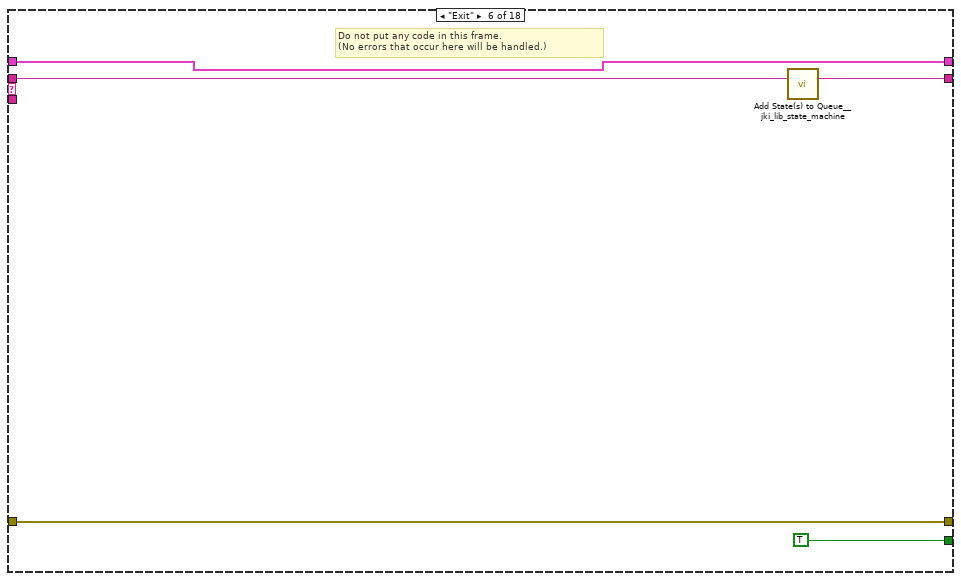
[diagram p8: hidden frame]
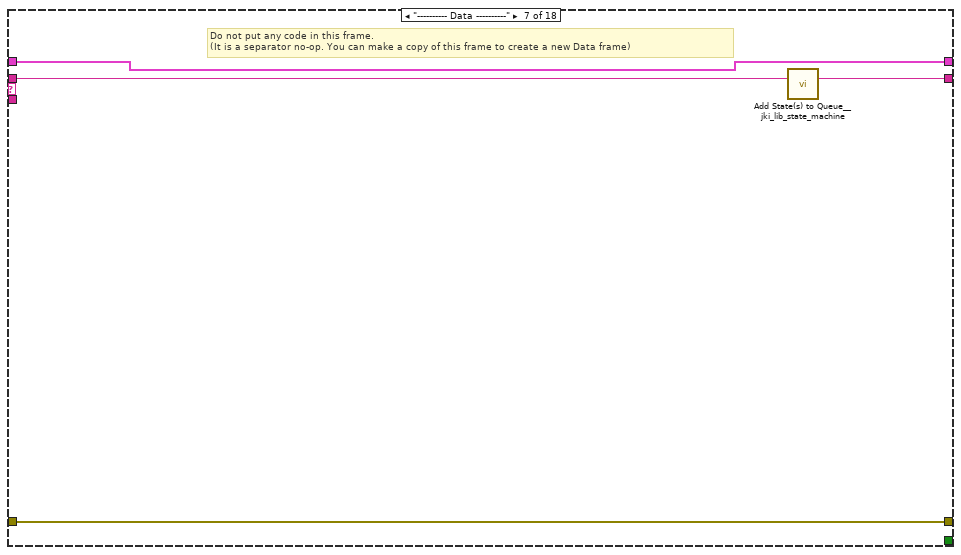
[diagram p9: hidden frame]
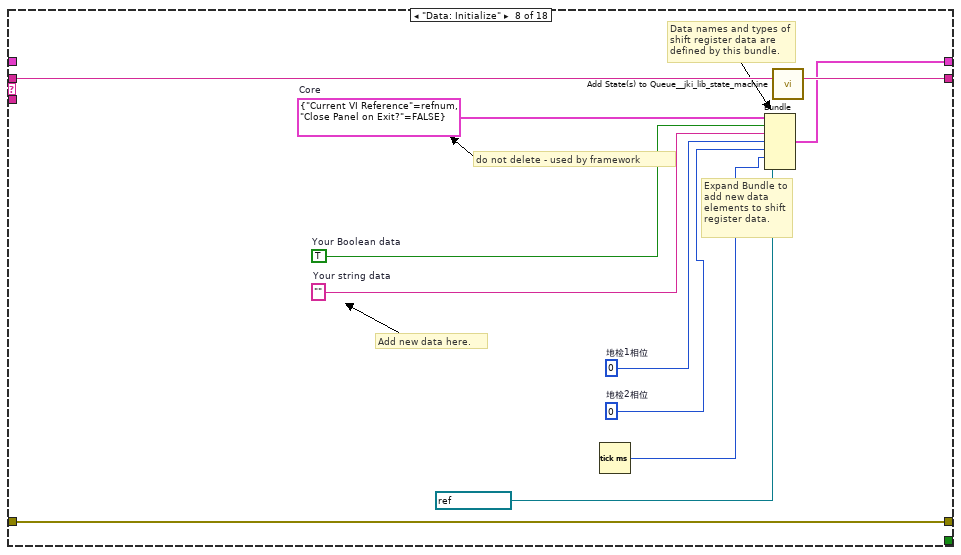
[diagram p10: hidden frame]
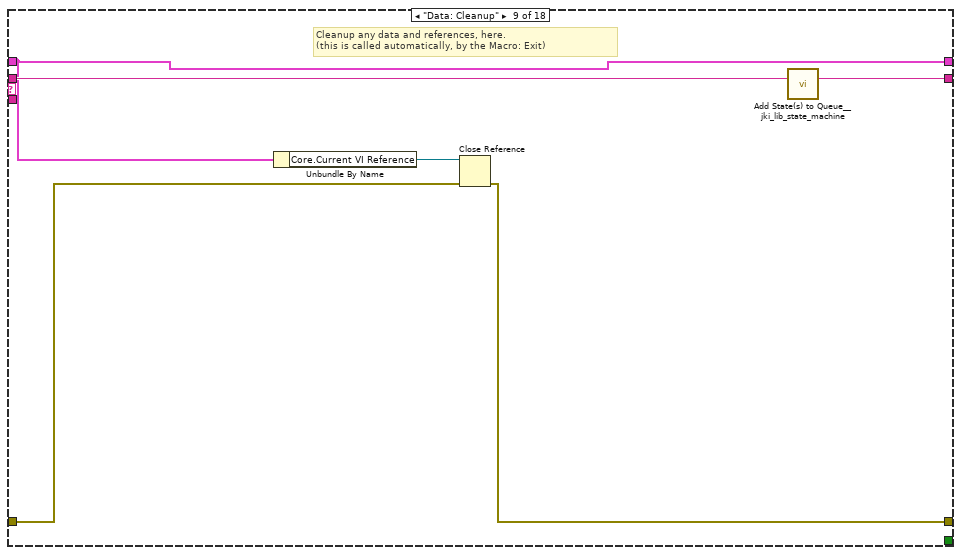
[diagram p11: hidden frame]
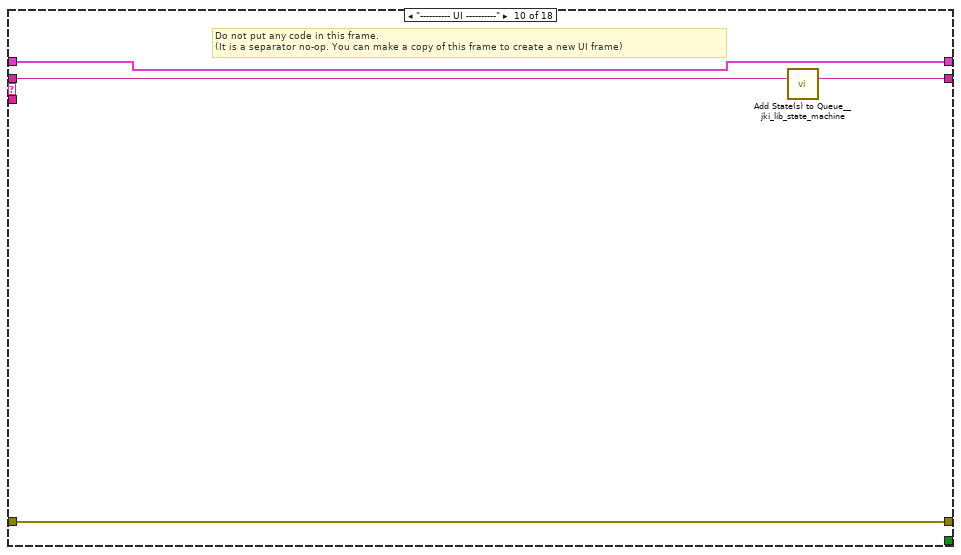
[diagram p12: hidden frame]
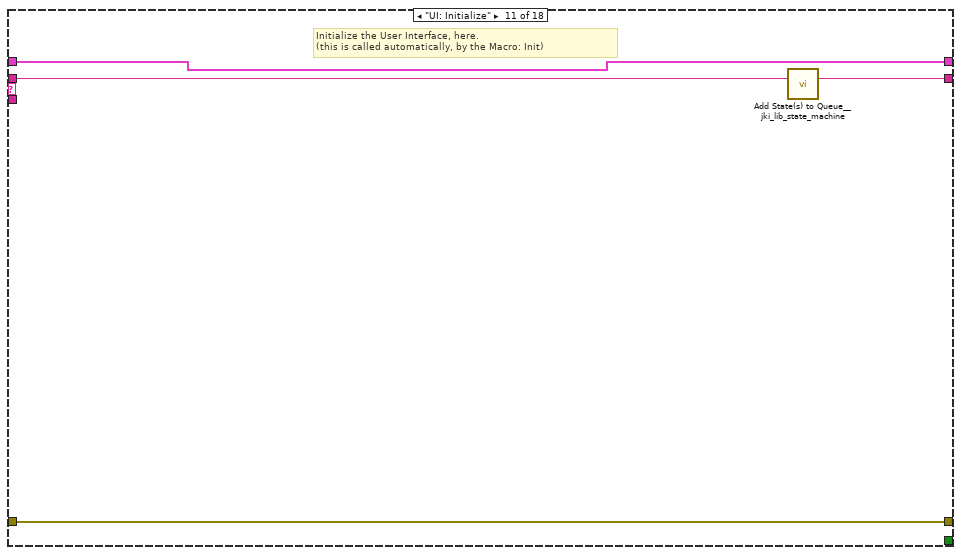
[diagram p13: hidden frame]
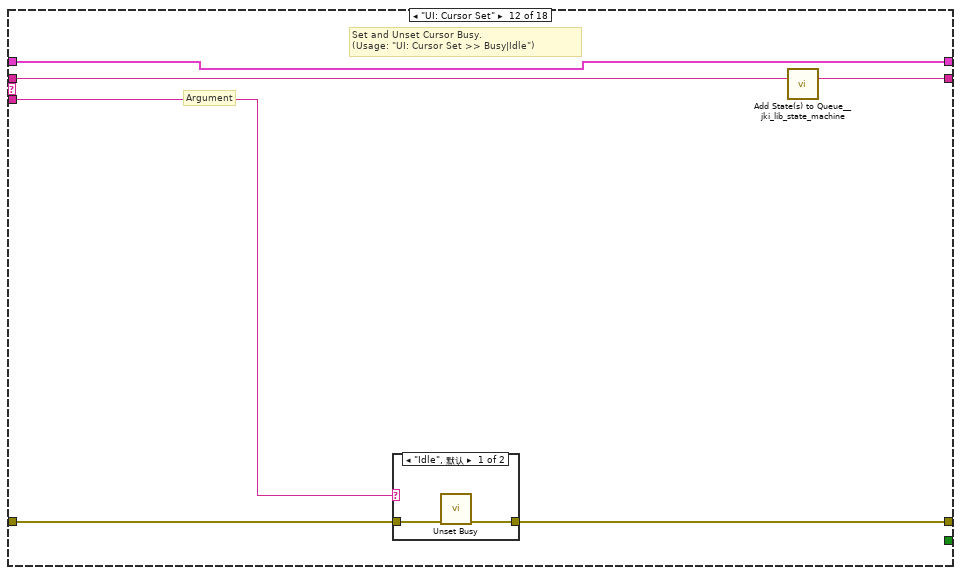
[diagram p14: hidden frame]
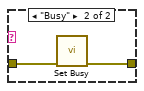
[diagram p15: hidden frame]
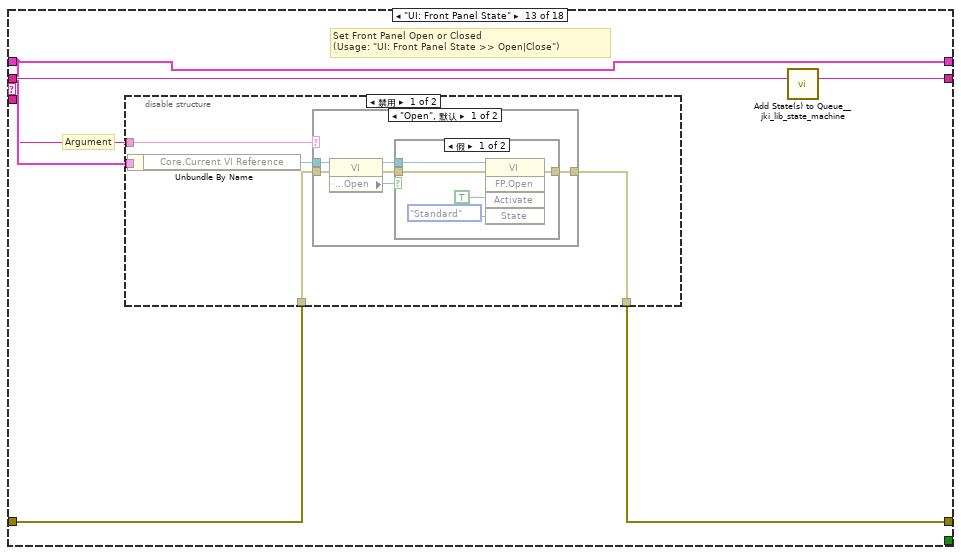
[diagram p16: hidden frame]
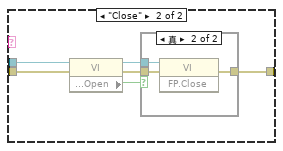
[diagram p18: hidden frame]
diagram:
  n1 = call <vilib>:"Add State(s) to Queue__jki_lib_state_machine.vi"("State(s) in (\"\")"="Macro: Initialize\nconfig:visa_Initialize\nconfig:zhufen\nconfig:beifen") -> ("States Out"=w6:string)  [unwired: 14 in]
  n2 = call <vilib>:"Add State(s) to Queue__jki_lib_state_machine.vi"("State(s) in (\"\")"="Macro: Initialize") -> ("States Out"=w3:string)  [unwired: 14 in]
  n3 = while "JKI - String-Based Queued State Machine (Basic) v1.0" {
    shift-right: [w13] -> _
    shift-left: _ -> [w12]
    shift-right: [w16] -> _
    shift-left: _ -> [w11]
    shift-right: [w15] -> _
    shift-left: w3 -> [w17]
    tunnel: "notifier" -> [w10]
    stop <- w14 stop-if-true
    n4 = call <vilib>:"Parse State Queue__jki_lib_state_machine.vi"("State Queue"=w17, "Error In (no error)"=w11) -> ("Remaining States"=w8:string, "Current State"=w19:string, "Arguments"=w18:string)  [unwired: 11 in]
    n5 = call "stop_message.vi"("notifier"=w10) -> ("通知"=w7:string)  [unwired: 9 in, 1 out]
    n6 = call <vilib>:"Add State(s) to Queue__jki_lib_state_machine.vi"("State(s) in (\"\")"=w8, "State(s) at Back (\"\")"=w7) -> ("States Out"=w9:string)  [unwired: 13 in]
    n7 = case shown="\"\", \"Idle\"" w19 {
      selector: w19 -> [_ _ w67 _ _ _ _ _ _ _ _ _ _ _ _ _ _ _]
      tunnel: w9 -> [w48 w66 w71 w89 w95 w100 w104 w115 w121 w125 w129 w135 w145 w176 w181 w191 w195 w200]
      tunnel: w18 -> [_ _ _ _ _ _ _ _ _ _ _ w130 w140 _ _ _ _ _]
      tunnel: w12 -> [w41 w63 w69 w80 w92 w98 w101 _ w116 w122 w127 w133 w141 w173 w178 w188 w192 w197]
      tunnel: [w20 w64 w73 w86 errorcluster {"status"=FALSE, "code"=0, "source"=""} ("error out") w97 w102 w112 w117 w123 w126 w131 w142 w174 w179 w189 w193 w198] -> w16
      tunnel: w11 -> [w23 w64 w72 w86 w91 w97 w102 w112 w118 w123 w126 w132 w143 w174 w179 w189 w193 w198]
      tunnel: [w47 w65 w70 w88 w94 w99 w103 w114 w120 w124 w128 w134 w144 w175 w180 w190 w194 w199] -> w15
      tunnel: [_ _ _ _ _ TRUE _ _ _ _ _ _ _ _ _ _ _ _] -> w14
      tunnel: [w40 w63 w69 w87 w92 w98 w101 w113 w116 w122 w127 w133 w141 w173 w178 w188 w192 w197] -> w13
      frame "", "Idle" {
        n8 = Unbundle By Name(w41) -> ("地检1相位"=w43:i32, "地检2相位"=w25:i32, "millisecond timer value"=w36:u32, "VISA资源名称"=w26:refnum<visa-resource-name>)
        n9 = Tick Count (ms)() -> (millisecond timer value=w37:u32)
        n10 = Subtract(x=w37, y=w36) -> (x-y=w39:u32)
        n11 = Greater Or Equal?(x=w39, y=u32 10) -> (x >= y?=w29:bool)
        n12 = call <vilib>:"Read.vi"("Register name"="DiJian_mode_Beifen") -> ("Register value"=w31:variant, "Error out"=w32:errorcluster)  [unwired: 11 in, 2 out]
        n13 = call <vilib>:"Read.vi"("Register name"="DiJian_mode") -> ("Register value"=w45:variant, "Error out"=w44:errorcluster)  [unwired: 11 in, 2 out]
        n14 = call-poly <vilib>:"Convert.vi"("Register value in"=w31, "Error in"=w32) -> ("Register value out"=w28:bool)  [unwired: 12 in, 1 out]
        n15 = call-poly <vilib>:"Convert.vi"("Register value in"=w45, "Error in"=w44) -> ("Register value out"=w34:bool)  [unwired: 12 in, 1 out]
        n16 = Select(t=w37, s=w29, f=w36) -> (s? t:f=w35:u32)
        n17 = And(x=w29, y=w28) -> (x .and. y?=w27:bool)
        n18 = And(x=w34, y=w29) -> (x .and. y?=w33:bool)
        n19 = case shown="真" w27 {
          tunnel: w26 -> [_ w55]
          tunnel: w25 -> [w50 w54]
          tunnel: [w50 w53] -> w24
          tunnel: w23 -> [w49 w52]
          tunnel: [w49 w51] -> w22
          frame False {
          }
          frame True {
            n20 = call "DiJian_2.vi"("error in"=w52, "地检2相位"=w54, "VISA资源名称"=w55) -> ("错误输出"=w51:errorcluster, "地检2相位输出"=w53:i32)  [unwired: 6 in, 1 out]
          }
        }
        n21 = case shown="真" w33 {
          tunnel: w43 -> [w57 w59]
          tunnel: [w57 w62] -> w42
          tunnel: w26 -> [_ w60]
          tunnel: w23 -> [w56 w58]
          tunnel: [w56 w61] -> w21
          frame False {
          }
          frame True {
            n22 = call "DiJian_1.vi"("error in"=w58, "地检1相位"=w59, "VISA资源名称"=w60) -> ("错误输出"=w61:errorcluster, "地检1相位输出"=w62:i32)  [unwired: 6 in, 1 out]
          }
        }
        n23 = Bundle By Name(cluster=w41, "地检1相位"=w42, "地检2相位"=w24, "millisecond timer value"=w35) -> (w40:T5)
        n24 = call <vilib>:"Add State(s) to Queue__jki_lib_state_machine.vi"("State(s) in (\"\")"=w48) -> ("States Out"=w47:string)  [unwired: 14 in]
        n25 = Merge Errors(w21, w22) -> (w20:errorcluster)
      }
      frame "---------- Core ----------" {
        # "Do not put any code in this frame.\n(it is a separator no-op)"
        n26 = call <vilib>:"Add State(s) to Queue__jki_lib_state_machine.vi"("State(s) in (\"\")"=w66) -> ("States Out"=w65:string)  [unwired: 14 in]
      }
      frame Default {
        w76 = 42 items=["No error", "Argument error", "Memory is full", "Out of zone", "End of file", "File already open", "Generic file I/O error", "File not found", "File permission error", "Disk is full", "Duplicate path", "Too many files open", "System feature not enabled", "Resource file not found", "Cannot add resource", "Resource not found", "Image not found", "Image memory error", "Pen does not exist", "Config type invalid", "Config token not found", "Config parse error", "Config memory error", "Bad external code format", "Bad external code offset", "External code not present", "Null window", "Destroy window error", "Null menu", "Print aborted", "Bad print record", "Print driver error", "Windows error during printing", "Memory error during printing", "Print dialog error", "Generic print error", "Invalid device refnum", "Device not found", "Device parameter error", "Device unit error", "Cannot open device", "Device call aborted", "Generic error", "Cancelled by user", "Object ID too low", "Object ID too high", "Object not in heap", "Unknown heap", "Unknown object (invalid DefProc)", "Unknown object (DefProc not in table)", "Message out of range", "Invalid (null) method", "Unknown message", "Manager call not supported", "Bad address", "Network operation in progress", "Network operation timed out", "Connection is busy", "Network attribute not supported", "Network error", "Address in use", "System out of memory", "Connection aborted", "Connection refused", "Not connected", "Already connected", "Connection closed", "Initialization error (interapplication manager)", "Bad occurrence", "Wait on unbound occurrence handler", "Occurrence queue overflow", "Datalog type conflict", "Unused", "Unrecognized type (interapplication manager)", "Memory corrupt", "Failed to make temporary DLL", "Old CIN version", "Drag socket not found", "Failed to load drop-object", "Failed to register OLE object", "Failed to release OLE object", "Format specifier type mismatch", "Unknown format specifier", "Too few format specifiers", "Too many format specifiers", "Scan failed", "Newer CIN version", "Error converting to variant", "Runtime menu error", "Password tampered", "Variant attribute not found", "Incompatible variant data type", "Event data is not available", "Event Store is not present", "Occurrence is not found", "Event Queue is not created", "Event info is not available", "Refnum passed is NULL", "Error retrieving Class GUID", "Error retrieving CoClass GUID", "Error retrieving TypeLib GUID.", "Bad built application magic bytes.", "Specific driver is different from the specific driver associated with the Logical Name.", "There is no session opened to the class driver.", "Max Error", "MAX - Error with config objects", "MAX - Error loading configuration", "MAX - Group not supported"]
        # "Current State"
        # "Do not delete, rename, or modify this frame.\n(this is used to capture unhandled states and typos)"
        # "Handle mistyped state name (developer tool)"
        n27 = Format Into String(format string="Software Exception: Unhandled State \"%s\"." ("message"), error in=w72, w67) -> (resulting string=w75:string, error out=w74:errorcluster)  [unwired: 1 in]
        n28 = call <vilib>:"Error Cluster From Error Code.vi"("show call chain? (False)"=TRUE, "error in (no error)"=w74, "error message (\"\")"=w75, "error code (0)"=w76) -> ("error out"=w73:errorcluster)  [unwired: 5 in]
        n29 = call <vilib>:"Add State(s) to Queue__jki_lib_state_machine.vi"("State(s) in (\"\")"=w71) -> ("States Out"=w70:string)  [unwired: 14 in]
      }
      frame "Initialize Core Data" {
        # "Do not delete, rename, or modify this frame.\n(this is used to determine panel behavior on exit)"
        # "originally closed?"
        # "exe?"
        # "If panel starts closed or is an EXE, then close it when we exit"
        n30 = property class="VI"() -> ("Front Panel.Open"=w85:bool)  [unwired: 2 in, 2 out]
        n31 = property class="App"() -> ("App.Kind"=w84:T3)  [unwired: 2 in, 2 out]
        n32 = control-ref of="Current VI Reference"() -> (w78:refnum<vi>)
        n33 = Not(x=w85) -> (.not. x?=w82:bool)
        n34 = Equal?(x=w84, y=T3."Run Time System" ("Application:Kind")) -> (x = y?=w81:bool)
        n35 = Or(x=w82, y=w81) -> (x .or. y?=w79:bool)
        n36 = Bundle By Name(cluster=w80, "Core.Current VI Reference"=w78, "Core.Close Panel on Exit?"=w79) -> (w87:T5)
        n37 = call <vilib>:"Add State(s) to Queue__jki_lib_state_machine.vi"("State(s) in (\"\")"=w89) -> ("States Out"=w88:string)  [unwired: 14 in]
      }
      frame "Error Handler" {
        # "Unhandled Error -- Display it"
        # "Handle any errors here.\nYou can also output any states to clean-up after errors occur"
        # "Clear error"
        n38 = call <vilib>:"General Error Handler.vi"("error in (no error)"=w91) -> ()  [unwired: 10 in, 5 out]
        n39 = call <vilib>:"Add State(s) to Queue__jki_lib_state_machine.vi"("State(s) in Front (\"\")"="/* Post Error States", "State(s) in (\"\")"=w95) -> ("States Out"=w94:string)  [unwired: 13 in]
      }
      frame "Exit" {
        # "Do not put any code in this frame.\n(No errors that occur here will be handled.)"
        n40 = call <vilib>:"Add State(s) to Queue__jki_lib_state_machine.vi"("State(s) in (\"\")"=w100) -> ("States Out"=w99:string)  [unwired: 14 in]
      }
      frame "---------- Data ----------" {
        # "Do not put any code in this frame.\n(It is a separator no-op. You can make a copy of this frame to create a new Data frame)"
        n41 = call <vilib>:"Add State(s) to Queue__jki_lib_state_machine.vi"("State(s) in (\"\")"=w104) -> ("States Out"=w103:string)  [unwired: 14 in]
      }
      frame "Data: Initialize" {
        w107 = 0  # 地检2相位
        w108 = 0  # 地检1相位
        w109 = T6 {"Current VI Reference"=refnum, "Close Panel on Exit?"=FALSE}  # Core
        w111 = TRUE  # Your Boolean data
        w110 = ""  # Your string data
        # "do not delete - used by framework"
        # "Expand Bundle to add new data elements to shift register data."
        # "Add new data here."
        # "Data names and types of shift register data are defined by this bundle."
        n42 = Tick Count (ms)() -> (millisecond timer value=w106:u32)
        n43 = Bundle("Core"=w109, "Your Boolean data"=w111, "Your string data"=w110, "地检1相位"=w108, "地检2相位"=w107, "millisecond timer value"=w106, "VISA资源名称"=refnum<visa-resource-name> "422_card") -> (w113:T5)  [unwired: 1 in]
        n44 = call <vilib>:"Add State(s) to Queue__jki_lib_state_machine.vi"("State(s) in (\"\")"=w115) -> ("States Out"=w114:string)  [unwired: 14 in]
      }
      frame "Data: Cleanup" {
        # "Cleanup any data and references, here.\n(this is called automatically, by the Macro: Exit)"
        n45 = Unbundle By Name(w116) -> ("Core.Current VI Reference"=w119:refnum<vi>)
        n46 = Close Reference(reference=w119, error in (no error)=w118) -> (error out=w117:errorcluster)
        n47 = call <vilib>:"Add State(s) to Queue__jki_lib_state_machine.vi"("State(s) in (\"\")"=w121) -> ("States Out"=w120:string)  [unwired: 14 in]
      }
      frame "---------- UI ----------" {
        # "Do not put any code in this frame.\n(It is a separator no-op. You can make a copy of this frame to create a new UI frame)"
        n48 = call <vilib>:"Add State(s) to Queue__jki_lib_state_machine.vi"("State(s) in (\"\")"=w125) -> ("States Out"=w124:string)  [unwired: 14 in]
      }
      frame "UI: Initialize" {
        # "Initialize the User Interface, here.\n(this is called automatically, by the Macro: Init)"
        n49 = call <vilib>:"Add State(s) to Queue__jki_lib_state_machine.vi"("State(s) in (\"\")"=w129) -> ("States Out"=w128:string)  [unwired: 14 in]
      }
      frame "UI: Cursor Set" {
        # "Argument"
        # "Set and Unset Cursor Busy.\n(Usage: \"UI: Cursor Set >> Busy|Idle\")"
        n50 = case shown="\"Idle\", 默认" w130 {
          tunnel: w132 -> [w137 w139]
          tunnel: [w136 w138] -> w131
          frame "Idle", Default {
            n51 = call <vilib>:"Unset Busy.vi"("error in (no error)"=w137) -> ("error out"=w136:errorcluster)  [unwired: 10 in]
          }
          frame "Busy" {
            n52 = call <vilib>:"Set Busy.vi"("error in (no error)"=w139) -> ("error out"=w138:errorcluster)  [unwired: 9 in, 1 out]
          }
        }
        n53 = call <vilib>:"Add State(s) to Queue__jki_lib_state_machine.vi"("State(s) in (\"\")"=w135) -> ("States Out"=w134:string)  [unwired: 14 in]
      }
      frame "UI: Front Panel State" {
        # "Argument"
        # "Set Front Panel Open or Closed\n(Usage: \"UI: Front Panel State >> Open|Close\")"
        n54 = disable-structure shown="禁用" {
          disable-tunnel: w143 -> [w150 _]
          disable-tunnel: [w149 _] -> w142
          disable-tunnel: w141 -> [w148 _]
          disable-tunnel: w140 -> [w146 _]
          frame Disabled {
            n55 = Unbundle By Name(w148) -> ("Core.Current VI Reference"=w147:refnum<vi>)
            n56 = case shown="\"Open\", 默认" w146 {
              tunnel: w150 -> [w154 w167]
              tunnel: [w156 w168] -> w149
              tunnel: w147 -> [w155 w165]
              frame "Open", Default {
                n57 = property class="VI"(reference=w155, error in=w154) -> (reference out=w152:refnum<vi>, error out=w153:errorcluster, "Front Panel.Open"=w151:bool)
                n58 = case shown="假" w151 {
                  tunnel: [w159 w162] -> w156
                  tunnel: w153 -> [w158 w162]
                  tunnel: w152 -> [w157 _]
                  frame False {
                    n59 = invoke class="VI" method="FP.Open"(reference=w157, error in=w158, "Activate"=TRUE, "State"=T4."Standard") -> (error out=w159:errorcluster)  [unwired: 1 in, 4 out]
                  }
                  frame True {
                  }
                }
              }
              frame "Close" {
                n60 = property class="VI"(reference=w165, error in=w167) -> (reference out=w164:refnum<vi>, error out=w166:errorcluster, "Front Panel.Open"=w163:bool)
                n61 = case shown="真" w163 {
                  tunnel: [w169 w172] -> w168
                  tunnel: w166 -> [w169 w171]
                  tunnel: w164 -> [_ w170]
                  frame False {
                  }
                  frame True {
                    n62 = invoke class="VI" method="FP.Close"(reference=w170, error in=w171) -> (error out=w172:errorcluster)  [unwired: 1 in, 2 out]
                  }
                }
              }
            }
          }
          frame Enabled {
          }
        }
        n63 = call <vilib>:"Add State(s) to Queue__jki_lib_state_machine.vi"("State(s) in (\"\")"=w145) -> ("States Out"=w144:string)  [unwired: 14 in]
      }
      frame "---------- Macro ----------" {
        # "Do not put any code in this frame.\n(It is a separator no-op. You can make a copy of this frame to create a new Macro frame)"
        n64 = call <vilib>:"Add State(s) to Queue__jki_lib_state_machine.vi"("State(s) in (\"\")"=w176) -> ("States Out"=w175:string)  [unwired: 14 in]
      }
      frame "Macro: Initialize" {
        w177 = "Data: Initialize\nInitialize Core Data\nUI: Initialize\nUI: Front Panel State >> Open"  # Data: Initialize Initialize Core Data UI: Initialize UI: Front Panel State >> Open
        # "Initialization Macro\n(This is called once, when the VI starts)"
        n65 = call <vilib>:"Add State(s) to Queue__jki_lib_state_machine.vi"("State(s) in Front (\"\")"=w177, "State(s) in (\"\")"=w181) -> ("States Out"=w180:string)  [unwired: 13 in]
      }
      frame "Macro: Exit" {
        # "Exit Macro\n(This is called once, when the VI exits)"
        n66 = Unbundle By Name(w188) -> ("Core.Close Panel on Exit?"=w187:bool)
        n67 = Select(t="UI: Front Panel State >> Close", s=w187, f="") -> (s? t:f=w184:string)
        n68 = call <vilib>:"Add State(s) to Queue__jki_lib_state_machine.vi"("State(s) in (\"\")"=w184, "State(s) at Back (\"\")"="Data: Cleanup\nExit") -> ("States Out"=w182:string)  [unwired: 13 in]
        n69 = call <vilib>:"Add State(s) to Queue__jki_lib_state_machine.vi"("State(s) in Front (\"\")"=w182, "State(s) in (\"\")"=w191) -> ("States Out"=w190:string)  [unwired: 13 in]
      }
      frame "---------- New Category ----------" {
        # "Template Separator\n(You can make a copy of, or modify, this frame)"
        n70 = call <vilib>:"Add State(s) to Queue__jki_lib_state_machine.vi"("State(s) in (\"\")"=w195) -> ("States Out"=w194:string)  [unwired: 14 in]
      }
      frame "Exit:all" {
        # "Exit:all"
        # "Your code here.\n(You can make a copy of, or modify, this frame)"
        n71 = call <vilib>:"Add State(s) to Queue__jki_lib_state_machine.vi"("State(s) in Front (\"\")"="Macro: Exit" ("State(s) in Front (\"\")"), "State(s) in (\"\")"=w200) -> ("States Out"=w199:string)  [unwired: 13 in]
      }
    }
  }
  n72 = while "JKI - String-Based Queued State Machine (Basic) v1.0" {
    shift-right: [w210] -> _
    shift-left: _ -> [w209]
    shift-right: [w212] -> _
    shift-left: _ -> [w208]
    shift-right: [w211] -> _
    shift-left: w6 -> [w213]
    tunnel: "notifier" -> [w201]
    tunnel: "传递队列" -> [w207]
    stop <- w206 stop-if-true
    n73 = call <vilib>:"Parse State Queue__jki_lib_state_machine.vi"("State Queue"=w213, "Error In (no error)"=w208) -> ("Remaining States"=w205:string, "Current State"=w215:string, "Arguments"=w214:string)  [unwired: 11 in]
    n74 = call "stop_message.vi"("识别符"="Cpci", "notifier"=w201) -> ("通知"=w203:string)  [unwired: 8 in, 1 out]
    n75 = call <vilib>:"Add State(s) to Queue__jki_lib_state_machine.vi"("State(s) in (\"\")"=w205, "State(s) at Back (\"\")"=w203) -> ("States Out"=w204:string)  [unwired: 13 in]
    n76 = case shown="\"config:zhufen\"" w215 {
      selector: w215 -> [_ _ w335 _ _ _ _ _ _ _ _ _ _ _ _ _ _ _ _ _ _ _ _ _ _ _ _ _ _ _ _ _ _ _ _ _ _ _ _]
      tunnel: w204 -> [w222 w334 w339 w357 w363 w368 w372 w388 w401 w408 w412 w418 w428 w460 w465 w475 w479 w488 w531 w548 w588 w634 w648 w660 w673 w677 w689 w702 w706 w717 w750 w784 w796 w809 w822 w826 w843 w851 w855]
      tunnel: w214 -> [_ _ _ _ _ _ _ _ _ _ _ w413 w423 _ _ _ _ _ _ _ w584 w603 _ _ _ _ _ _ _ _ _ _ _ _ _ _ _ _ _]
      tunnel: w209 -> [w218 w331 w337 w348 w360 w366 w369 _ w399 w405 w410 w416 w424 w457 w462 w472 w476 w480 w514 w536 w586 w632 w645 w651 w670 w674 w680 w699 w703 w709 w742 w780 w792 w807 w820 w823 w838 w848 w856]
      tunnel: [w227 w332 w341 w354 errorcluster {"status"=FALSE, "code"=0, "source"=""} ("error out") w365 w370 w374 w398 w406 w409 w414 w425 w458 w463 w473 w477 w486 w529 w533 w556 w599 w646 w649 w663 w675 w678 w692 w704 w710 w743 w778 w790 w797 w812 w824 w827 w849 w852] -> w212
      tunnel: w208 -> [w226 w332 w340 w354 w359 w365 w370 w383 w396 w406 w409 w415 w426 w458 w463 w473 w477 w485 w515 _ w579 w627 w646 w655 w667 w675 w684 w696 w704 w712 w745 w775 w785 w803 w810 w824 w828 w849 w852]
      tunnel: [w221 w333 w338 w356 w362 w367 w371 w387 w400 w407 w411 w417 w427 w459 w464 w474 w478 w487 w530 w547 w587 w633 w647 w659 w672 w676 w688 w701 w705 w716 w749 w783 w795 w808 w821 w825 w842 w850 w854] -> w211
      tunnel: [w217 w331 w337 w355 w360 w366 w369 w386 w399 w405 w410 w416 w424 w457 w462 w472 w476 w480 w514 w535 w586 w632 w645 w651 w670 w674 w680 w699 w703 w709 w742 w780 w792 w807 w820 w823 w838 w848 w856] -> w210
      tunnel: w207 -> [w225 _ _ _ _ _ _ _ _ _ _ _ _ _ _ _ _ _ _ _ _ _ _ _ _ _ _ _ _ _ _ _ _ _ _ _ _ _ _]
      tunnel: [_ _ _ _ _ TRUE _ _ _ _ _ _ _ _ _ _ _ _ _ _ _ _ _ _ _ _ _ _ _ _ _ _ _ _ _ _ _ _ _] -> w206
      tunnel: w201 -> [_ _ _ _ _ _ _ w373 _ _ _ _ _ _ _ _ _ _ _ _ _ _ _ _ _ _ _ _ _ _ _ _ _ _ _ _ _ _ _]
      frame "", "Idle" {
        n77 = Dequeue Element(queue=w225, timeout in ms (-1)=1 ("超时毫秒(-1)"), error in (no error)=w226) -> (element=w224:T9, timed out?=w219:bool, error out=w223:errorcluster)  [unwired: 1 out]
        n78 = case shown="真" w219 {
          tunnel: [w239 w299] -> w227
          tunnel: w218 -> [w229 w310]
          tunnel: w224 -> [w238 _]
          tunnel: w223 -> [w237 w302]
          tunnel: [w230 w309] -> w217
          tunnel: [w228 "" ("State(s) at Back (\"\")")] -> w216
          frame False {
            n79 = Unbundle By Name(w238) -> ("数据帧名称"=w232:string, "数据"=w231:string, "读写标志"=w236:i32)
            n80 = Unbundle By Name(w229) -> ("visa"=w235:refnum<visa-resource-name>[])
            n81 = Index Array(array=w235) -> (element=w233:refnum<visa-resource-name>)  [unwired: 1 in]
            n82 = String To Byte Array(string=w231) -> (unsigned byte array=w234:u8[])
            n83 = case shown="\"1553B_CMD_Zhufen\", 默认" w232 {
              tunnel: w237 -> [w247 w269 w294]
              tunnel: [w246 w268 w294] -> w239
              tunnel: w236 -> [w245 w267 _]
              tunnel: w233 -> [w244 w266 _]
              tunnel: w234 -> [w243 w265 _]
              tunnel: w231 -> [w240 w263 w293]
              tunnel: w229 -> [w242 w264 w290]
              tunnel: [w242 w264 w285] -> w230
              tunnel: [w241 w262 "Run:switch chanelA_B" ("State(s) at Back (\"\")")] -> w228
              frame "1553B_CMD_Zhufen", Default {
                n84 = case shown="2" w245 {
                  tunnel: w247 -> [w252 w259 w261]
                  tunnel: [w249 w259 w261] -> w246
                  tunnel: w244 -> [w254 _ _]
                  tunnel: w243 -> [w253 _ _]
                  tunnel: ["" ("State(s) at Back (\"\")") w255 "" ("State(s) at Back (\"\")")] -> w241
                  tunnel: w240 -> [_ w257 _]
                  frame 1 {
                    n85 = call "1553B_Msg.vi"("Timeout(默认:5ms)"=5, "error in"=w252, "主备份选择"=enum8{"主份", "备份"}."主份", "unsigned byte array"=w253, "VISA资源名称"=w254) -> ("error out 2"=w249:errorcluster)  [unwired: 4 in, 2 out]
                  }
                  frame 2 {
                    # "1为控制指令，2为通用寄存器配置"
                    n86 = Concatenate Strings("config:period_zhufen" ("State(s) at Back (\"\")"), ">>" ("字符串"), w257) -> (w255:string)
                  }
                  frame 3, Default {
                  }
                }
              }
              frame "1553B_CMD_Beifen" {
                n87 = case shown="2" w267 {
                  tunnel: w269 -> [w271 w281 w282]
                  tunnel: [w274 w281 w282] -> w268
                  tunnel: w266 -> [w272 _ _]
                  tunnel: w265 -> [w273 _ _]
                  tunnel: w263 -> [_ w278 _]
                  tunnel: ["" w277 ""] -> w262
                  frame 1 {
                    n88 = call "1553B_Msg.vi"("Timeout(默认:5ms)"=5, "error in"=w271, "主备份选择"=enum8{"主份", "备份"}."备份", "unsigned byte array"=w273, "VISA资源名称"=w272) -> ("error out 2"=w274:errorcluster)  [unwired: 4 in, 2 out]
                  }
                  frame 2 {
                    n89 = Concatenate Strings("config:period_beifen" ("State(s) at Back (\"\")"), ">>" ("字符串"), w278) -> (w277:string)
                  }
                  frame 3, Default {
                  }
                }
              }
              frame "SwitchChanel" {
                n90 = Unflatten From String(type=T7 {"主份通道选择"=enum."通道A", "备份通道选择"=enum."通道B"} ("输入簇"), binary string=w293) -> (value=w291:T7)  [unwired: 3 in, 2 out]
                n91 = Unbundle By Name(w291) -> ("主份通道选择"=w289:enum32{"通道A", "通道B"}, "备份通道选择"=w287:enum32{"通道A", "通道B"})
                n92 = case shown="\"通道A\", 默认" w287 {
                  tunnel: [enum8{"ChanleA", "ChanelB"}."ChanleA" ("主份通道选择") enum8{"ChanleA", "ChanelB"}."ChanelB" ("主份通道选择")] -> w286
                  frame "通道A", Default {
                  }
                  frame "通道B" {
                  }
                }
                n93 = case shown="\"通道A\", 默认" w289 {
                  tunnel: [enum8{"ChanleA", "ChanelB"}."ChanleA" ("主份通道选择") enum8{"ChanleA", "ChanelB"}."ChanelB" ("主份通道选择")] -> w288
                  frame "通道A", Default {
                  }
                  frame "通道B" {
                  }
                }
                n94 = Bundle By Name(cluster=w290, "主份通道选择"=w288, "备份通道选择"=w286) -> (w285:T8)
              }
            }
          }
          frame True {
            n95 = Unbundle By Name(w310) -> ("visa"=w322:refnum<visa-resource-name>[], "毫秒计时值"=w312:u32)
            n96 = Tick Count (ms)() -> (millisecond timer value=w313:u32)
            n97 = Subtract(x=w313, y=w312) -> (x-y=w315:u32)
            n98 = Greater Or Equal?(x=w315, y=u32 5) -> (x >= y?=w304:bool)
            n99 = call <vilib>:"Read.vi"("Register name"="Zhufen_on") -> ("Register value"=w318:variant)  [unwired: 11 in, 3 out]
            n100 = Select(t=w313, s=w304, f=w312) -> (s? t:f=w311:u32)
            n101 = call <vilib>:"Read.vi"("Register name"="Beifen_on") -> ("Register value"=w307:variant)  [unwired: 11 in, 3 out]
            n102 = call-poly <vilib>:"Convert.vi"("Register value in"=w318) -> ("Register value out"=w317:bool)  [unwired: 13 in, 1 out]
            n103 = Index Array(array=w322, index=0 ("索引")) -> (element=w305:refnum<visa-resource-name>)
            n104 = Bundle By Name(cluster=w310, "毫秒计时值"=w311) -> (w309:T8)
            n105 = call-poly <vilib>:"Convert.vi"("Register value in"=w307) -> ("Register value out"=w308:bool)  [unwired: 13 in, 1 out]
            n106 = And(x=w304, y=w317) -> (x .and. y?=w316:bool)
            n107 = And(x=w304, y=w308) -> (x .and. y?=w303:bool)
            n108 = case shown="真" w316 {
              tunnel: w302 -> [w327 w329]
              tunnel: [w327 w328] -> w301
              tunnel: w305 -> [_ w330]
              frame False {
              }
              frame True {
                n109 = call "1553B_RECV_fifo.vi"("错误输入（无错误）"=w329, "VISA资源名称输入"=w330) -> ("error out 2"=w328:errorcluster)  [unwired: 8 in, 1 out]
              }
            }
            n110 = case shown="真" w303 {
              tunnel: [w323 w325] -> w300
              tunnel: w305 -> [_ w324]
              tunnel: w302 -> [w323 w326]
              frame False {
              }
              frame True {
                n111 = call "1553B_Recv-Beifen.vi"("错误输入（无错误）"=w326, "VISA资源名称输入"=w324) -> ("error out 2"=w325:errorcluster)  [unwired: 8 in, 1 out]
              }
            }
            n112 = Merge Errors(w301, w300) -> (w299:errorcluster)
          }
        }
        n113 = call <vilib>:"Add State(s) to Queue__jki_lib_state_machine.vi"("State(s) in (\"\")"=w222, "State(s) at Back (\"\")"=w216) -> ("States Out"=w221:string)  [unwired: 13 in]
      }
      frame "---------- Core ----------" {
        n114 = call <vilib>:"Add State(s) to Queue__jki_lib_state_machine.vi"("State(s) in (\"\")"=w334) -> ("States Out"=w333:string)  [unwired: 14 in]
      }
      frame Default {
        w344 = 42 items=["No error", "Argument error", "Memory is full", "Out of zone", "End of file", "File already open", "Generic file I/O error", "File not found", "File permission error", "Disk is full", "Duplicate path", "Too many files open", "System feature not enabled", "Resource file not found", "Cannot add resource", "Resource not found", "Image not found", "Image memory error", "Pen does not exist", "Config type invalid", "Config token not found", "Config parse error", "Config memory error", "Bad external code format", "Bad external code offset", "External code not present", "Null window", "Destroy window error", "Null menu", "Print aborted", "Bad print record", "Print driver error", "Windows error during printing", "Memory error during printing", "Print dialog error", "Generic print error", "Invalid device refnum", "Device not found", "Device parameter error", "Device unit error", "Cannot open device", "Device call aborted", "Generic error", "Cancelled by user", "Object ID too low", "Object ID too high", "Object not in heap", "Unknown heap", "Unknown object (invalid DefProc)", "Unknown object (DefProc not in table)", "Message out of range", "Invalid (null) method", "Unknown message", "Manager call not supported", "Bad address", "Network operation in progress", "Network operation timed out", "Connection is busy", "Network attribute not supported", "Network error", "Address in use", "System out of memory", "Connection aborted", "Connection refused", "Not connected", "Already connected", "Connection closed", "Initialization error (interapplication manager)", "Bad occurrence", "Wait on unbound occurrence handler", "Occurrence queue overflow", "Datalog type conflict", "Unused", "Unrecognized type (interapplication manager)", "Memory corrupt", "Failed to make temporary DLL", "Old CIN version", "Drag socket not found", "Failed to load drop-object", "Failed to register OLE object", "Failed to release OLE object", "Format specifier type mismatch", "Unknown format specifier", "Too few format specifiers", "Too many format specifiers", "Scan failed", "Newer CIN version", "Error converting to variant", "Runtime menu error", "Password tampered", "Variant attribute not found", "Incompatible variant data type", "Event data is not available", "Event Store is not present", "Occurrence is not found", "Event Queue is not created", "Event info is not available", "Refnum passed is NULL", "Error retrieving Class GUID", "Error retrieving CoClass GUID", "Error retrieving TypeLib GUID.", "Bad built application magic bytes.", "Specific driver is different from the specific driver associated with the Logical Name.", "There is no session opened to the class driver.", "Max Error", "MAX - Error with config objects", "MAX - Error loading configuration", "MAX - Group not supported"]
        # "Current State"
        # "Do not delete, rename, or modify this frame.\n(this is used to capture unhandled states and typos)"
        # "Handle mistyped state name (developer tool)"
        n115 = Format Into String(format string="Software Exception: Unhandled State \"%s\"." ("message"), error in=w340, w335) -> (resulting string=w343:string, error out=w342:errorcluster)  [unwired: 1 in]
        n116 = call <vilib>:"Error Cluster From Error Code.vi"("show call chain? (False)"=TRUE, "error in (no error)"=w342, "error message (\"\")"=w343, "error code (0)"=w344) -> ("error out"=w341:errorcluster)  [unwired: 5 in]
        n117 = call <vilib>:"Add State(s) to Queue__jki_lib_state_machine.vi"("State(s) in (\"\")"=w339) -> ("States Out"=w338:string)  [unwired: 14 in]
      }
      frame "Initialize Core Data" {
        # "Do not delete, rename, or modify this frame.\n(this is used to determine panel behavior on exit)"
        # "originally closed?"
        # "exe?"
        # "If panel starts closed or is an EXE, then close it when we exit"
        n118 = property class="VI"() -> ("Front Panel.Open"=w353:bool)  [unwired: 2 in, 2 out]
        n119 = property class="App"() -> ("App.Kind"=w352:T3)  [unwired: 2 in, 2 out]
        n120 = control-ref of="Current VI Reference"() -> (w346:refnum<vi>)
        n121 = Not(x=w353) -> (.not. x?=w350:bool)
        n122 = Equal?(x=w352, y=T3."Run Time System" ("Application:Kind")) -> (x = y?=w349:bool)
        n123 = Or(x=w350, y=w349) -> (x .or. y?=w347:bool)
        n124 = Bundle By Name(cluster=w348, "Core.Current VI Reference"=w346, "Core.Close Panel on Exit?"=w347) -> (w355:T8)
        n125 = call <vilib>:"Add State(s) to Queue__jki_lib_state_machine.vi"("State(s) in (\"\")"=w357) -> ("States Out"=w356:string)  [unwired: 14 in]
      }
      frame "Error Handler" {
        # "Unhandled Error -- Display it"
        # "Handle any errors here.\nYou can also output any states to clean-up after errors occur"
        # "Clear error"
        n126 = call <vilib>:"General Error Handler.vi"("error in (no error)"=w359) -> ()  [unwired: 10 in, 5 out]
        n127 = call <vilib>:"Add State(s) to Queue__jki_lib_state_machine.vi"("State(s) in Front (\"\")"="/* Post Error States", "State(s) in (\"\")"=w363) -> ("States Out"=w362:string)  [unwired: 13 in]
      }
      frame "Exit" {
        n128 = call <vilib>:"Add State(s) to Queue__jki_lib_state_machine.vi"("State(s) in (\"\")"=w368) -> ("States Out"=w367:string)  [unwired: 14 in]
      }
      frame "---------- Data ----------" {
        # "Do not put any code in this frame.\n(It is a separator no-op. You can make a copy of this frame to create a new Data frame)"
        n129 = call <vilib>:"Add State(s) to Queue__jki_lib_state_machine.vi"("State(s) in (\"\")"=w372) -> ("States Out"=w371:string)  [unwired: 14 in]
      }
      frame "Data: Initialize" {
        w380 = enum8{"ChanleA", "ChanelB"}."ChanleA"  # 备份通道选择
        w381 = enum8{"ChanleA", "ChanelB"}."ChanleA"  # 主份通道选择
        w385 = T6 {"Current VI Reference"=refnum, "Close Panel on Exit?"=FALSE}  # Core
        n130 = for {
          tunnel: refnum<visa-resource-name>[] ["422_card", "OC_card", "AI_card"] ("资源名称") -> [w392] mode=indexing
          tunnel: [w391] -> w382 mode=indexing
          shift-right: [w389] -> w375
          shift-left: w383 -> [w390]
          n131 = VISA Open(error in (no error)=w390, VISA resource name=w392) -> (VISA resource name=w391:refnum<visa-resource-name>, error out=w389:errorcluster)  [unwired: 3 in]
        }
        n132 = Tick Count (ms)() -> (millisecond timer value=w379:u32)
        n133 = Bundle(cluster=T8 {"Core"={"Current VI Reference"=refnum, "Close Panel on Exit?"=FALSE}, "visa"=[], "主份通道选择"=enum."ChanleA", "备份通道选择"=enum."ChanleA", "毫秒计时值"=0, "notifier "=refnum} ("输出簇"), "Core"=w385, "visa"=w382, "主份通道选择"=w381, "备份通道选择"=w380, "毫秒计时值"=w379, "notifier"=w373) -> (w386:T8)
        n134 = call <vilib>:"Add State(s) to Queue__jki_lib_state_machine.vi"("State(s) in (\"\")"=w388) -> ("States Out"=w387:string)  [unwired: 14 in]
        n135 = call <vilib>:"Write.vi"("Register name"="DiJian_mode", "Register value"=FALSE, "Error in"=w375) -> ("Error out"=w374:errorcluster)  [unwired: 10 in, 2 out]
      }
      frame "Data: Cleanup" {
        n136 = Unbundle By Name(w399) -> ("visa"=w394:refnum<visa-resource-name>[], "Core.Current VI Reference"=w395:refnum<vi>)
        n137 = Index Array(array=w394) -> (element=w393:refnum<visa-resource-name>)  [unwired: 1 in]
        n138 = call "DisInterrupt.vi"("InstrHandle"=w393) -> ()  [unwired: 9 in, 2 out]
        n139 = Close Reference(reference=w395, error in (no error)=w396) -> (error out=w397:errorcluster)
        n140 = for {
          shift-right: [w403] -> w398
          shift-left: w397 -> [w404]
          tunnel: w394 -> [w402] mode=indexing
          n141 = VISA Close(VISA resource name=w402, error in (no error)=w404) -> (error out=w403:errorcluster)
        }
        n142 = call <vilib>:"Add State(s) to Queue__jki_lib_state_machine.vi"("State(s) in (\"\")"=w401) -> ("States Out"=w400:string)  [unwired: 14 in]
      }
      frame "---------- UI ----------" {
        # "Do not put any code in this frame.\n(It is a separator no-op. You can make a copy of this frame to create a new UI frame)"
        n143 = call <vilib>:"Add State(s) to Queue__jki_lib_state_machine.vi"("State(s) in (\"\")"=w408) -> ("States Out"=w407:string)  [unwired: 14 in]
      }
      frame "UI: Initialize" {
        # "Initialize the User Interface, here.\n(this is called automatically, by the Macro: Init)"
        n144 = call <vilib>:"Add State(s) to Queue__jki_lib_state_machine.vi"("State(s) in (\"\")"=w412) -> ("States Out"=w411:string)  [unwired: 14 in]
      }
      frame "UI: Cursor Set" {
        # "Argument"
        # "Set and Unset Cursor Busy.\n(Usage: \"UI: Cursor Set >> Busy|Idle\")"
        n145 = case shown="\"Idle\", 默认" w413 {
          tunnel: w415 -> [w420 w422]
          tunnel: [w419 w421] -> w414
          frame "Idle", Default {
            n146 = call <vilib>:"Unset Busy.vi"("error in (no error)"=w420) -> ("error out"=w419:errorcluster)  [unwired: 10 in]
          }
          frame "Busy" {
            n147 = call <vilib>:"Set Busy.vi"("error in (no error)"=w422) -> ("error out"=w421:errorcluster)  [unwired: 9 in, 1 out]
          }
        }
        n148 = call <vilib>:"Add State(s) to Queue__jki_lib_state_machine.vi"("State(s) in (\"\")"=w418) -> ("States Out"=w417:string)  [unwired: 14 in]
      }
      frame "UI: Front Panel State" {
        # "Set Front Panel Open or Closed\n(Usage: \"UI: Front Panel State >> Open|Close\")"
        n149 = disable-structure shown="启用" {
          disable-tunnel: w426 -> [w433 w456]
          disable-tunnel: [w432 w456] -> w425
          disable-tunnel: w424 -> [w431 _]
          disable-tunnel: w423 -> [w429 _]
          frame Disabled {
            # "Argument"
            n150 = Unbundle By Name(w431) -> ("Core.Current VI Reference"=w430:refnum<vi>)
            n151 = case shown="\"Close\"" w429 {
              tunnel: w433 -> [w437 w450]
              tunnel: [w439 w451] -> w432
              tunnel: w430 -> [w438 w448]
              frame "Open", Default {
                n152 = property class="VI"(reference=w438, error in=w437) -> (reference out=w435:refnum<vi>, error out=w436:errorcluster, "Front Panel.Open"=w434:bool)
                n153 = case shown="假" w434 {
                  tunnel: [w442 w445] -> w439
                  tunnel: w436 -> [w441 w445]
                  tunnel: w435 -> [w440 _]
                  frame False {
                    n154 = invoke class="VI" method="FP.Open"(reference=w440, error in=w441, "Activate"=TRUE, "State"=T4."Standard") -> (error out=w442:errorcluster)  [unwired: 1 in, 4 out]
                  }
                  frame True {
                  }
                }
              }
              frame "Close" {
                n155 = property class="VI"(reference=w448, error in=w450) -> (reference out=w447:refnum<vi>, error out=w449:errorcluster, "Front Panel.Open"=w446:bool)
                n156 = case shown="真" w446 {
                  tunnel: [w452 w455] -> w451
                  tunnel: w449 -> [w452 w454]
                  tunnel: w447 -> [_ w453]
                  frame False {
                  }
                  frame True {
                    n157 = invoke class="VI" method="FP.Close"(reference=w453, error in=w454) -> (error out=w455:errorcluster)  [unwired: 1 in, 2 out]
                  }
                }
              }
            }
          }
          frame Enabled {
          }
        }
        n158 = call <vilib>:"Add State(s) to Queue__jki_lib_state_machine.vi"("State(s) in (\"\")"=w428) -> ("States Out"=w427:string)  [unwired: 14 in]
      }
      frame "---------- Macro ----------" {
        # "Do not put any code in this frame.\n(It is a separator no-op. You can make a copy of this frame to create a new Macro frame)"
        n159 = call <vilib>:"Add State(s) to Queue__jki_lib_state_machine.vi"("State(s) in (\"\")"=w460) -> ("States Out"=w459:string)  [unwired: 14 in]
      }
      frame "Macro: Initialize" {
        # "Initialization Macro\n(This is called once, when the VI starts)"
        n160 = call <vilib>:"Add State(s) to Queue__jki_lib_state_machine.vi"("State(s) in Front (\"\")"="Data: Initialize\nInitialize Core Data\nUI: Initialize\nUI: Front Panel State >> Close\n\n", "State(s) in (\"\")"=w465) -> ("States Out"=w464:string)  [unwired: 13 in]
      }
      frame "Macro: Exit" {
        # "Exit Macro\n(This is called once, when the VI exits)"
        n161 = Unbundle By Name(w472) -> ("Core.Close Panel on Exit?"=w471:bool)
        n162 = Select(t="UI: Front Panel State >> Close", s=w471, f="") -> (s? t:f=w468:string)
        n163 = call <vilib>:"Add State(s) to Queue__jki_lib_state_machine.vi"("State(s) in (\"\")"=w468, "State(s) at Back (\"\")"="Data: Cleanup\nExit") -> ("States Out"=w466:string)  [unwired: 13 in]
        n164 = call <vilib>:"Add State(s) to Queue__jki_lib_state_machine.vi"("State(s) in Front (\"\")"=w466, "State(s) in (\"\")"=w475) -> ("States Out"=w474:string)  [unwired: 13 in]
      }
      frame "---------- Config ----------" {
        # "Template Separator\n(You can make a copy of, or modify, this frame)"
        n165 = call <vilib>:"Add State(s) to Queue__jki_lib_state_machine.vi"("State(s) in (\"\")"=w479) -> ("States Out"=w478:string)  [unwired: 14 in]
      }
      frame "config:visa_Initialize" {
        n166 = Unbundle By Name(w480) -> ("visa"=w483:refnum<visa-resource-name>[])
        n167 = for {
          N: 1 -> [_]
          tunnel: [w491] -> _ mode=indexing
          shift-right: [w490] -> w486
          shift-left: w485 -> [w495]
          tunnel: w483 -> [w494] mode=indexing
          tunnel: "8路定时配置 2" -> [w493] mode=indexing
          tunnel: "8路通用配置" -> [w492] mode=indexing
          # "硬件定时模式"
          n168 = for {
            N: 8 -> [_]
            shift-right: [w500] -> w490
            shift-left: w495 -> [w501]
            shift-right: [w498] -> w491
            shift-left: w494 -> [w499]
            tunnel: w493 -> [w497] mode=indexing
            tunnel: w492 -> [w496] mode=indexing
            i -> [w507]
            n169 = To Unsigned Long Integer(number=w507) -> (unsigned 32bit integer=w510:u32)
            n170 = Multiply(x=w510, y=u32 1048576 ("基地址")) -> (x*y=w509:u32)
            n171 = Add(x=u32 1048624 ("基地址"), y=w509) -> (x+y=w503:u32)
            n172 = Add(x=u32 1048580 ("基地址"), y=w509) -> (x+y=w506:u32)
            n173 = call "通用参数设置.vi"("通用寄存器配置输入"=w496) -> ("通用寄存器配置输出"=w508:u32[])  [unwired: 10 in]
            n174 = call-poly <vilib>:"write.vi"("error out"=w501, "起始地址"=w506, "U32"=w508, "VISA资源名称输入"=w499) -> ("error out 2"=w502:errorcluster, "VISA资源名称输出"=w505:refnum<visa-resource-name>)  [unwired: 6 in]
            n175 = call "硬件定时参数设置.vi"("硬件定时配置输入"=w497) -> ("硬件定时配置输出"=w504:u32[])  [unwired: 10 in]
            n176 = call-poly <vilib>:"write.vi"("error out"=w502, "起始地址"=w503, "U32"=w504, "VISA资源名称输入"=w505) -> ("error out 2"=w500:errorcluster, "VISA资源名称输出"=w498:refnum<visa-resource-name>)  [unwired: 6 in]
          }
        }
        n177 = call <vilib>:"Add State(s) to Queue__jki_lib_state_machine.vi"("State(s) in (\"\")"=w488) -> ("States Out"=w487:string)  [unwired: 14 in]
      }
      frame "config:zhufen" {
        n178 = Unbundle By Name(w514) -> ("visa"=w518:refnum<visa-resource-name>[])
        n179 = Index Array(array=w518) -> (element=w517:refnum<visa-resource-name>)  [unwired: 1 in]
        n180 = call "1553B_Msg_cirle.vi"("error in"=w515, "主备份选择"=enum8{"主份", "备份"}."主份", "VISA资源名称"=w517) -> ("error out 2"=w529:errorcluster, "VISAout"=w522:refnum<visa-resource-name>)  [unwired: 6 in, 1 out]
        n181 = call-poly <vilib>:"write.vi"("起始地址"=u32 3145864 ("基地址"), "U32"=u32[] [8388608, 256], "VISA资源名称输入"=w522) -> ("VISA资源名称输出"=w521:refnum<visa-resource-name>)  [unwired: 7 in, 1 out]
        n182 = call-poly <vilib>:"write.vi"("起始地址"=u32 3145936 ("基地址"), "U32"=u32[] [65536], "VISA资源名称输入"=w521) -> ("VISA资源名称输出"=w524:refnum<visa-resource-name>)  [unwired: 7 in, 1 out]
        n183 = call-poly <vilib>:"write.vi"("起始地址"=u32 48 ("基地址"), "U32"=u32[] [24], "VISA资源名称输入"=w524) -> ("VISA资源名称输出"=w523:refnum<visa-resource-name>)  [unwired: 7 in, 1 out]
        n184 = call "EnInterrupt.vi"("InstrHandle"=w523) -> ()  [unwired: 9 in, 2 out]
        n185 = call <vilib>:"Add State(s) to Queue__jki_lib_state_machine.vi"("State(s) in (\"\")"=w531) -> ("States Out"=w530:string)  [unwired: 14 in]
      }
      frame "config:beifen" {
        n186 = Unbundle By Name(w536) -> ("visa"=w539:refnum<visa-resource-name>[])
        n187 = Index Array(array=w539) -> (element=w541:refnum<visa-resource-name>)  [unwired: 1 in]
        n188 = call "1553B_Msg_cirle.vi"("主备份选择"=enum8{"主份", "备份"}."备份", "VISA资源名称"=w541) -> ("error out 2"=w538:errorcluster, "VISAout"=w545:refnum<visa-resource-name>)  [unwired: 7 in, 1 out]
        n189 = call-poly <vilib>:"write.vi"("error out"=w538, "起始地址"=u32 4194440 ("基地址"), "U32"=u32[] [8388608, 256], "VISA资源名称输入"=w545) -> ("error out 2"=w537:errorcluster, "VISA资源名称输出"=w544:refnum<visa-resource-name>)  [unwired: 6 in]
        n190 = call-poly <vilib>:"write.vi"("error out"=w537, "起始地址"=u32 4194512 ("基地址"), "U32"=u32[] [65536], "VISA资源名称输入"=w544) -> ("error out 2"=w534:errorcluster)  [unwired: 6 in, 1 out]
        n191 = flat-sequence {
          tunnel: w536 -> [w552]
          tunnel: [w550] -> w535
          tunnel: w534 -> [w549]
          tunnel: [w549] -> w533
          frame #0 {
            n192 = Tick Count (ms)() -> (millisecond timer value=w551:u32)
            n193 = Bundle By Name(cluster=w552, "毫秒计时值"=w551) -> (w550:T8)
          }
        }
        n194 = call <vilib>:"Add State(s) to Queue__jki_lib_state_machine.vi"("State(s) in (\"\")"=w548) -> ("States Out"=w547:string)  [unwired: 14 in]
      }
      frame "config:period_zhufen" {
        w571 = u32 3145836 ("偏移量(0)")
        n195 = Unbundle By Name(w586) -> ("visa"=w585:refnum<visa-resource-name>[])
        n196 = Decimal String To Number(string=w584) -> (number=w554:i32)  [unwired: 2 in, 1 out]
        n197 = Index Array(array=w585) -> (element=w580:refnum<visa-resource-name>)  [unwired: 1 in]
        n198 = To Unsigned Long Integer(number=w554) -> (unsigned 32bit integer=w583:u32)
        n199 = case shown="160, 默认" w554 {
          tunnel: [u16[] [52224] ("数据字数组") u16[] [49920] ("数据字数组")] -> w553
          frame 160, Default {
          }
          frame 480 {
          }
        }
        n200 = Decrement(x=w583) -> (x-1=w578:u32)
        n201 = Build Array(w578) -> (w581:u32[])
        n202 = call "1553B_CMD_Sync.vi"("数据字数组"=w553) -> ("1553B指令"=w558:string)  [unwired: 10 in]
        n203 = call-poly <vilib>:"write.vi"("error out"=w579, "起始地址"=u32 3145860 ("偏移量(0)"), "U32"=w581, "VISA资源名称输入"=w580) -> ("error out 2"=w557:errorcluster, "VISA资源名称输出"=w555:refnum<visa-resource-name>)  [unwired: 6 in]
        n204 = call "Cpci_Read.vi"("u32_len"=1, "基地址"=w571, "VISA资源名称"=w555) -> ("U8"=w560:u8[], "VISA资源名称输出"=w569:refnum<visa-resource-name>)  [unwired: 6 in, 1 out]
        n205 = Reverse 1D Array(array=w560) -> (reversed array=w559:u8[])
        n206 = String To Byte Array(string=w558) -> (unsigned byte array=w572:u8[])
        n207 = Type Cast(type=u32 1 ("u32_len"), x=w559) -> (*(type *) &x=w566:u32)
        n208 = Array Size(array=w572) -> (size(s)=w576:i32)
        n209 = To Unsigned Long Integer(number=w576) -> (unsigned 32bit integer=w564:u32)
        n210 = And(x=w566, y=u32 65535) -> (x .and. y?=w565:u32)
        n211 = Logical Shift(y=i16 16, x=w564) -> (x << y=w562:u32)
        n212 = Add(x=w562, y=w565) -> (x+y=w563:u32)
        "x+y" <- w563
        n213 = Build Array(w563) -> (w575:u32[])
        n214 = Wait (ms)(milliseconds to wait=u32 1 ("等待时间（毫秒）")) -> ()  [unwired: 1 out]
        n215 = call-poly <vilib>:"write.vi"("error out"=w557, "起始地址"=w571, "U32"=w575, "VISA资源名称输入"=w569) -> ("error out 2"=w574:errorcluster, "VISA资源名称输出"=w573:refnum<visa-resource-name>)  [unwired: 6 in]
        n216 = disable-structure shown="启用" {
          disable-tunnel: w574 -> [w595 w597]
          disable-tunnel: [w594 w597] -> w556
          disable-tunnel: w573 -> [w593 w598]
          disable-tunnel: w572 -> [w592 _]
          disable-tunnel: [w591 w598] -> _
          frame Enabled {
            n217 = call-poly <vilib>:"write.vi"("error out"=w595, "起始地址"=u32 3146368 ("偏移量(0)"), "数组"=w592, "VISA资源名称输入"=w593) -> ("error out 2"=w594:errorcluster, "VISA资源名称 输出"=w591:refnum<visa-resource-name>)  [unwired: 6 in]
          }
          frame Disabled {
          }
        }
        n218 = call <vilib>:"Add State(s) to Queue__jki_lib_state_machine.vi"("State(s) in (\"\")"=w588) -> ("States Out"=w587:string)  [unwired: 14 in]
      }
      frame "config:period_beifen" {
        w618 = u32 4194412 ("偏移量(0)")
        n219 = Unbundle By Name(w632) -> ("visa"=w631:refnum<visa-resource-name>[])
        n220 = Index Array(array=w631) -> (element=w628:refnum<visa-resource-name>)  [unwired: 1 in]
        n221 = Decimal String To Number(string=w603) -> (number=w601:i32)  [unwired: 2 in, 1 out]
        n222 = case shown="480" w601 {
          tunnel: [u16[] [52224] ("数据字数组") u16[] [49920] ("数据字数组")] -> w604
          frame 160, Default {
          }
          frame 480 {
          }
        }
        n223 = To Unsigned Long Integer(number=w601) -> (unsigned 32bit integer=w626:u32)
        n224 = Decrement(x=w626) -> (x-1=w625:u32)
        n225 = Build Array(w625) -> (w629:u32[])
        n226 = call-poly <vilib>:"write.vi"("error out"=w627, "起始地址"=u32 4194436 ("偏移量(0)"), "U32"=w629, "VISA资源名称输入"=w628) -> ("error out 2"=w600:errorcluster, "VISA资源名称输出"=w602:refnum<visa-resource-name>)  [unwired: 6 in]
        n227 = call "Cpci_Read.vi"("u32_len"=1, "基地址"=w618, "VISA资源名称"=w602) -> ("U8"=w607:u8[], "VISA资源名称输出"=w616:refnum<visa-resource-name>)  [unwired: 6 in, 1 out]
        n228 = Reverse 1D Array(array=w607) -> (reversed array=w606:u8[])
        n229 = call "1553B_CMD_Sync.vi"("数据字数组"=w604) -> ("1553B指令"=w605:string)  [unwired: 10 in]
        n230 = String To Byte Array(string=w605) -> (unsigned byte array=w619:u8[])
        n231 = Type Cast(type=u32 1 ("u32_len"), x=w606) -> (*(type *) &x=w613:u32)
        n232 = Array Size(array=w619) -> (size(s)=w623:i32)
        n233 = To Unsigned Long Integer(number=w623) -> (unsigned 32bit integer=w611:u32)
        n234 = And(x=w613, y=u32 65535) -> (x .and. y?=w612:u32)
        n235 = Logical Shift(y=i16 16, x=w611) -> (x << y=w609:u32)
        n236 = Add(x=w609, y=w612) -> (x+y=w610:u32)
        "x+y 2" <- w610
        n237 = Build Array(w610) -> (w622:u32[])
        n238 = Wait (ms)(milliseconds to wait=u32 1 ("等待时间（毫秒）")) -> ()  [unwired: 1 out]
        n239 = call <vilib>:"Add State(s) to Queue__jki_lib_state_machine.vi"("State(s) in (\"\")"=w634) -> ("States Out"=w633:string)  [unwired: 14 in]
        n240 = call-poly <vilib>:"write.vi"("error out"=w600, "起始地址"=w618, "U32"=w622, "VISA资源名称输入"=w616) -> ("error out 2"=w621:errorcluster, "VISA资源名称输出"=w620:refnum<visa-resource-name>)  [unwired: 6 in]
        n241 = disable-structure shown="启用" {
          disable-tunnel: w621 -> [w641 w643]
          disable-tunnel: [w640 w643] -> w599
          disable-tunnel: w620 -> [w639 w644]
          disable-tunnel: w619 -> [w638 _]
          disable-tunnel: [w637 w644] -> _
          frame Enabled {
            n242 = call-poly <vilib>:"write.vi"("error out"=w641, "起始地址"=u32 4194944 ("偏移量(0)"), "数组"=w638, "VISA资源名称输入"=w639) -> ("error out 2"=w640:errorcluster, "VISA资源名称 输出"=w637:refnum<visa-resource-name>)  [unwired: 6 in]
          }
          frame Disabled {
          }
        }
      }
      frame "---------- Zhufen--------" {
        n243 = call <vilib>:"Add State(s) to Queue__jki_lib_state_machine.vi"("State(s) in (\"\")"=w648) -> ("States Out"=w647:string)  [unwired: 14 in]
      }
      frame "Zhufen:stop" {
        n244 = Unbundle By Name(w651) -> ("visa"=w658:refnum<visa-resource-name>[])
        n245 = Index Array(array=w658) -> (element=w654:refnum<visa-resource-name>)  [unwired: 1 in]
        n246 = call-poly <vilib>:"write.vi"("error out"=w655, "起始地址"=u32 3145776 ("偏移量(0)"), "U32"=u32[] [0], "VISA资源名称输入"=w654) -> ("error out 2"=w650:errorcluster)  [unwired: 6 in, 1 out]
        n247 = Unbundle By Name(w651) -> ("notifier"=w652:refnum<notifier>)
        n248 = Send Notification(notification="SaveFileTxt__Zhufen:stop" ("通知"), notifier=w652, error in (no error)=w650) -> (error out=w649:errorcluster)  [unwired: 1 out]
        n249 = call <vilib>:"Add State(s) to Queue__jki_lib_state_machine.vi"("State(s) in (\"\")"=w660) -> ("States Out"=w659:string)  [unwired: 14 in]
      }
      frame "Zhufen:CPCI_start" {
        n250 = Unbundle By Name(w670) -> ("visa"=w671:refnum<visa-resource-name>[])
        n251 = Index Array(array=w671) -> (element=w666:refnum<visa-resource-name>)  [unwired: 1 in]
        n252 = call-poly <vilib>:"write.vi"("error out"=w667, "起始地址"=u32 3145776 ("偏移量(0)"), "U32"=u32[] [131584], "VISA资源名称输入"=w666) -> ("error out 2"=w665:errorcluster, "VISA资源名称输出"=w664:refnum<visa-resource-name>)  [unwired: 6 in]
        n253 = call-poly <vilib>:"write.vi"("error out"=w665, "起始地址"=u32 3146884 ("偏移量(0)"), "U32"=u32[] [1], "VISA资源名称输入"=w664) -> ("error out 2"=w663:errorcluster)  [unwired: 6 in, 1 out]
        n254 = call <vilib>:"Add State(s) to Queue__jki_lib_state_machine.vi"("State(s) in (\"\")"=w673) -> ("States Out"=w672:string)  [unwired: 14 in]
      }
      frame "---------- Beifen--------" {
        n255 = call <vilib>:"Add State(s) to Queue__jki_lib_state_machine.vi"("State(s) in (\"\")"=w677) -> ("States Out"=w676:string)  [unwired: 14 in]
      }
      frame "Beifen:stop" {
        n256 = Unbundle By Name(w680) -> ("visa"=w687:refnum<visa-resource-name>[])
        n257 = Index Array(array=w687) -> (element=w683:refnum<visa-resource-name>)  [unwired: 1 in]
        n258 = call-poly <vilib>:"write.vi"("error out"=w684, "起始地址"=u32 4194352 ("偏移量(0)"), "U32"=u32[] [0], "VISA资源名称输入"=w683) -> ("error out 2"=w679:errorcluster)  [unwired: 6 in, 1 out]
        n259 = Unbundle By Name(w680) -> ("notifier"=w681:refnum<notifier>)
        n260 = Send Notification(notification="SaveFileTxt__Beifen:stop" ("通知"), notifier=w681, error in (no error)=w679) -> (error out=w678:errorcluster)  [unwired: 1 out]
        n261 = call <vilib>:"Add State(s) to Queue__jki_lib_state_machine.vi"("State(s) in (\"\")"=w689) -> ("States Out"=w688:string)  [unwired: 14 in]
      }
      frame "Beifen:CPCI_start" {
        n262 = Unbundle By Name(w699) -> ("visa"=w700:refnum<visa-resource-name>[])
        n263 = Index Array(array=w700) -> (element=w695:refnum<visa-resource-name>)  [unwired: 1 in]
        n264 = call-poly <vilib>:"write.vi"("error out"=w696, "起始地址"=u32 4194352 ("偏移量(0)"), "U32"=u32[] [131584], "VISA资源名称输入"=w695) -> ("error out 2"=w694:errorcluster, "VISA资源名称输出"=w693:refnum<visa-resource-name>)  [unwired: 6 in]
        n265 = call-poly <vilib>:"write.vi"("error out"=w694, "起始地址"=u32 4195460 ("偏移量(0)"), "U32"=u32[] [1], "VISA资源名称输入"=w693) -> ("error out 2"=w692:errorcluster)  [unwired: 6 in, 1 out]
        n266 = call <vilib>:"Add State(s) to Queue__jki_lib_state_machine.vi"("State(s) in (\"\")"=w702) -> ("States Out"=w701:string)  [unwired: 14 in]
      }
      frame "---------- Dijian--------" {
        n267 = call <vilib>:"Add State(s) to Queue__jki_lib_state_machine.vi"("State(s) in (\"\")"=w706) -> ("States Out"=w705:string)  [unwired: 14 in]
      }
      frame "DiJian:start" {
        n268 = Unbundle By Name(w709) -> ("visa"=w714:refnum<visa-resource-name>[])
        n269 = Index Array(array=w714) -> (element=w713:refnum<visa-resource-name>)  [unwired: 1 in]
        n270 = for {
          N: 2 -> [_]
          tunnel: w713 -> [w736]
          tunnel: w712 -> [w733]
          tunnel: [w730] -> w711
          i -> [w727]
          n271 = disable-structure shown="启用" {
            disable-tunnel: [u32[] [131584] ("U32") u32[] [1] ("U32")] -> w737
            frame Disabled {
            }
            frame Enabled {
            }
          }
          n272 = To Unsigned Long Integer(number=w727) -> (unsigned 32bit integer=w725:u32)
          n273 = Multiply(x=u32 1048576 ("偏移量(0)"), y=w725) -> (x*y=w720:u32)
          n274 = Add(x=u32 1048624 ("偏移量(0)"), y=w720) -> (x+y=w718:u32)
          n275 = Add(x=u32 1049868 ("偏移量(0)"), y=w720) -> (x+y=w722:u32)
          n276 = Add(x=u32 1049864 ("偏移量(0)"), y=w720) -> (x+y=w723:u32)
          n277 = call-poly <vilib>:"write.vi"("error out"=w733, "起始地址"=w723, "U32"=w737, "VISA资源名称输入"=w736) -> ("error out 2"=w732:errorcluster, "VISA资源名称输出"=w735:refnum<visa-resource-name>)  [unwired: 6 in]
          n278 = call-poly <vilib>:"write.vi"("error out"=w732, "起始地址"=w722, "U32"=u32[] [1], "VISA资源名称输入"=w735) -> ("error out 2"=w731:errorcluster, "VISA资源名称输出"=w729:refnum<visa-resource-name>)  [unwired: 6 in]
          n279 = call-poly <vilib>:"write.vi"("error out"=w731, "起始地址"=w718, "U32"=u32[] [2], "VISA资源名称输入"=w729) -> ("error out 2"=w730:errorcluster)  [unwired: 6 in, 1 out]
        }
        n280 = call <vilib>:"Write.vi"("Register name"="DiJian_mode", "Register value"=TRUE, "Error in"=w711) -> ("Error out"=w710:errorcluster)  [unwired: 10 in, 2 out]
        n281 = call <vilib>:"Add State(s) to Queue__jki_lib_state_machine.vi"("State(s) in (\"\")"=w717) -> ("States Out"=w716:string)  [unwired: 14 in]
      }
      frame "DiJian:start_Beifen" {
        n282 = Unbundle By Name(w742) -> ("visa"=w747:refnum<visa-resource-name>[])
        n283 = Index Array(array=w747) -> (element=w746:refnum<visa-resource-name>)  [unwired: 1 in]
        n284 = for {
          N: 2 -> [_]
          tunnel: w746 -> [w769]
          tunnel: w745 -> [w766]
          tunnel: [w763] -> w744
          i -> [w760]
          n285 = disable-structure shown="启用" {
            disable-tunnel: [u32[] [131584] ("U32") u32[] [1] ("U32")] -> w770
            frame Disabled {
            }
            frame Enabled {
            }
          }
          n286 = To Unsigned Long Integer(number=w760) -> (unsigned 32bit integer=w758:u32)
          n287 = Multiply(x=u32 2097152 ("偏移量(0)"), y=w758) -> (x*y=w753:u32)
          n288 = Add(x=u32 2097200 ("偏移量(0)"), y=w753) -> (x+y=w751:u32)
          n289 = Add(x=u32 2098444 ("偏移量(0)"), y=w753) -> (x+y=w755:u32)
          n290 = Add(x=u32 2098440 ("偏移量(0)"), y=w753) -> (x+y=w756:u32)
          n291 = call-poly <vilib>:"write.vi"("error out"=w766, "起始地址"=w756, "U32"=w770, "VISA资源名称输入"=w769) -> ("error out 2"=w765:errorcluster, "VISA资源名称输出"=w768:refnum<visa-resource-name>)  [unwired: 6 in]
          n292 = call-poly <vilib>:"write.vi"("error out"=w765, "起始地址"=w755, "U32"=u32[] [1], "VISA资源名称输入"=w768) -> ("error out 2"=w764:errorcluster, "VISA资源名称输出"=w762:refnum<visa-resource-name>)  [unwired: 6 in]
          n293 = call-poly <vilib>:"write.vi"("error out"=w764, "起始地址"=w751, "U32"=u32[] [2], "VISA资源名称输入"=w762) -> ("error out 2"=w763:errorcluster)  [unwired: 6 in, 1 out]
        }
        n294 = call <vilib>:"Write.vi"("Register name"="DiJian_mode_Beifen", "Register value"=TRUE, "Error in"=w744) -> ("Error out"=w743:errorcluster)  [unwired: 10 in, 2 out]
        n295 = call <vilib>:"Add State(s) to Queue__jki_lib_state_machine.vi"("State(s) in (\"\")"=w750) -> ("States Out"=w749:string)  [unwired: 14 in]
      }
      frame "DiJian:stop" {
        n296 = Unbundle By Name(w780) -> ("visa"=w779:refnum<visa-resource-name>[])
        n297 = Index Array(array=w779) -> (element=w774:refnum<visa-resource-name>)  [unwired: 1 in]
        n298 = call-poly <vilib>:"write.vi"("error out"=w775, "起始地址"=u32 1048624 ("偏移量(0)"), "U32"=u32[] [0], "VISA资源名称输入"=w774) -> ("error out 2"=w773:errorcluster)  [unwired: 6 in, 1 out]
        n299 = call <vilib>:"Write.vi"("Register name"="DiJian_mode", "Register value"=FALSE, "Error in"=w773) -> ("Error out"=w778:errorcluster)  [unwired: 10 in, 2 out]
        n300 = call <vilib>:"Add State(s) to Queue__jki_lib_state_machine.vi"("State(s) in (\"\")"=w784) -> ("States Out"=w783:string)  [unwired: 14 in]
      }
      frame "DiJian:stop_Beifen" {
        n301 = Unbundle By Name(w792) -> ("visa"=w791:refnum<visa-resource-name>[])
        n302 = Index Array(array=w791) -> (element=w786:refnum<visa-resource-name>)  [unwired: 1 in]
        n303 = call-poly <vilib>:"write.vi"("error out"=w785, "起始地址"=u32 2097200 ("偏移量(0)"), "U32"=u32[] [0], "VISA资源名称输入"=w786) -> ("error out 2"=w787:errorcluster)  [unwired: 6 in, 1 out]
        n304 = call <vilib>:"Write.vi"("Register name"="DiJian_mode_Beifen", "Register value"=FALSE, "Error in"=w787) -> ("Error out"=w790:errorcluster)  [unwired: 10 in, 2 out]
        n305 = call <vilib>:"Add State(s) to Queue__jki_lib_state_machine.vi"("State(s) in (\"\")"=w796) -> ("States Out"=w795:string)  [unwired: 14 in]
      }
      frame "DiJian:pause" {
        n306 = Unbundle By Name(w807) -> ("visa"=w806:refnum<visa-resource-name>[])
        n307 = Index Array(array=w806) -> (element=w802:refnum<visa-resource-name>)  [unwired: 1 in]
        n308 = call-poly <vilib>:"write.vi"("error out"=w803, "起始地址"=u32 1049876 ("偏移量(0)"), "U32"=u32[] [3], "VISA资源名称输入"=w802) -> ("error out 2"=w800:errorcluster, "VISA资源名称输出"=w801:refnum<visa-resource-name>)  [unwired: 6 in]
        n309 = call-poly <vilib>:"write.vi"("error out"=w800, "起始地址"=u32 1049872 ("偏移量(0)"), "U32"=u32[] [1], "VISA资源名称输入"=w801) -> ("error out 2"=w797:errorcluster)  [unwired: 6 in, 1 out]
        n310 = call <vilib>:"Add State(s) to Queue__jki_lib_state_machine.vi"("State(s) in (\"\")"=w809) -> ("States Out"=w808:string)  [unwired: 14 in]
      }
      frame "DiJian:pause_Beifen" {
        n311 = Unbundle By Name(w820) -> ("visa"=w819:refnum<visa-resource-name>[])
        n312 = Index Array(array=w819) -> (element=w811:refnum<visa-resource-name>)  [unwired: 1 in]
        n313 = call-poly <vilib>:"write.vi"("error out"=w810, "起始地址"=u32 2098452 ("偏移量(0)"), "U32"=u32[] [3], "VISA资源名称输入"=w811) -> ("error out 2"=w816:errorcluster, "VISA资源名称输出"=w815:refnum<visa-resource-name>)  [unwired: 6 in]
        n314 = call-poly <vilib>:"write.vi"("error out"=w816, "起始地址"=u32 2098448 ("偏移量(0)"), "U32"=u32[] [1], "VISA资源名称输入"=w815) -> ("error out 2"=w812:errorcluster)  [unwired: 6 in, 1 out]
        n315 = call <vilib>:"Add State(s) to Queue__jki_lib_state_machine.vi"("State(s) in (\"\")"=w822) -> ("States Out"=w821:string)  [unwired: 14 in]
      }
      frame "---------- Run ----------" {
        # "Template Separator\n(You can make a copy of, or modify, this frame)"
        n316 = call <vilib>:"Add State(s) to Queue__jki_lib_state_machine.vi"("State(s) in (\"\")"=w826) -> ("States Out"=w825:string)  [unwired: 14 in]
      }
      frame "Run:switch chanelA_B" {
        n317 = Unbundle By Name(w838) -> ("visa"=w841:refnum<visa-resource-name>[], "主份通道选择"=w835:enum8{"ChanleA", "ChanelB"}, "备份通道选择"=w834:enum8{"ChanleA", "ChanelB"})
        n318 = case shown="\"ChanleA\", 默认" w834 {
          tunnel: [u8[] [36, 67, 65, 5, 10] ("unsigned byte array") u8[] [36, 67, 66, 5, 10] ("unsigned byte array")] -> w830
          frame "ChanleA", Default {
          }
          frame "ChanelB" {
          }
        }
        n319 = case shown="\"ChanleA\", 默认" w835 {
          tunnel: [u8[] [36, 67, 65, 5, 10] ("unsigned byte array") u8[] [36, 67, 66, 5, 10] ("unsigned byte array")] -> w836
          frame "ChanleA", Default {
          }
          frame "ChanelB" {
          }
        }
        n320 = Index Array(array=w841) -> (element=w839:refnum<visa-resource-name>)  [unwired: 1 in]
        n321 = call "1553B_Msg.vi"("Timeout(默认:5ms)"=5, "error in"=w828, "主备份选择"=enum8{"主份", "备份"}."主份", "unsigned byte array"=w836, "VISA资源名称"=w839) -> ("error out 2"=w829:errorcluster, "VISAout"=w831:refnum<visa-resource-name>)  [unwired: 4 in, 1 out]
        n322 = call "1553B_Msg.vi"("Timeout(默认:5ms)"=5, "error in"=w829, "主备份选择"=enum8{"主份", "备份"}."备份", "unsigned byte array"=w830, "VISA资源名称"=w831) -> ("error out 2"=w827:errorcluster)  [unwired: 4 in, 2 out]
        n323 = call <vilib>:"Add State(s) to Queue__jki_lib_state_machine.vi"("State(s) in (\"\")"=w843) -> ("States Out"=w842:string)  [unwired: 14 in]
      }
      frame "-------- Exit--------" {
        # "Template Separator\n(You can make a copy of, or modify, this frame)"
        n324 = call <vilib>:"Add State(s) to Queue__jki_lib_state_machine.vi"("State(s) in (\"\")"=w851) -> ("States Out"=w850:string)  [unwired: 14 in]
      }
      frame "Exit:all" {
        n325 = call <vilib>:"Add State(s) to Queue__jki_lib_state_machine.vi"("State(s) in Front (\"\")"="Macro: Exit" ("State(s) in Front (\"\")"), "State(s) in (\"\")"=w855) -> ("States Out"=w854:string)  [unwired: 13 in]
      }
    }
  }
  n326 = while {
    tunnel: "notifier" -> [w861]
    stop <- w860 stop-if-true
    n327 = call "stop_message.vi"("notifier"=w861) -> ("Exit？"=w860:bool)  [unwired: 9 in, 1 out]
    n328 = call "Cpci_Read.vi"("u32_len"=9, "基地址"=u32 1048592, "VISA资源名称"=refnum<visa-resource-name> "AI_card") -> ("U8"=w862:u8[])  [unwired: 6 in, 2 out]
    n329 = Wait Until Next ms Multiple(millisecond multiple=u32 200 ("毫秒倍数")) -> ()  [unwired: 1 out]
    n330 = for {
      N: 9 -> [_]
      tunnel: w862 -> [w879]
      tunnel: [w872] -> w857 mode=indexing
      i -> [w871]
      n331 = Multiply(x=4, y=w871) -> (x*y=w877:i32)
      n332 = Array Subset(array=w879, index=w877, length=4 ("长度")) -> (w875:u8[])
      n333 = Reverse 1D Array(array=w875) -> (reversed array=w874:u8[])
      n334 = Type Cast(type=u32 14793 ("x"), x=w874) -> (*(type *) &x=w880:u32)
      n335 = Multiply(x=w880, y=24.576) -> (x*y=w886:dbl)
      n336 = Equal To 0?(x=w871) -> (x = 0?=w870:bool)
      n337 = Divide(x=w886, y=65536.0) -> (x/y=w884:dbl)
      n338 = Select(t=1.51 ("y"), s=w870, f=1.51 ("y")) -> (s? t:f=w867:dbl)
      n339 = Subtract(x=w884, y=12.288) -> (x-y=w882:dbl)
      n340 = Multiply(x=w882, y=w867) -> (x*y=w873:dbl)
      n341 = To Single Precision Float(number=w873) -> (single precision float=w872:sgl)
    }
    n342 = call <vilib>:"Write.vi"("Register name"="AIs", "Register value"=w857) -> ()  [unwired: 11 in, 3 out]
  }
